vi "Argos_K_0v85.vi"(0 "PID 1 COM":refnum<visa-resource-name>="COM1", 1 "Setpoint\n START":bool, 2 "Write to File":bool, 3 "SP 1 input (°C)":dbl=20.0 min=0.0 max=1300.0, 4 "Intervall (s)":u32=1 max=600, 5 "Write/\nRead":bool=TRUE, 6 "Delay (ms)":u32=500 min=100 max=600000, 7 "Auto Tune":bool, 9 "Standby":bool, 11 "Reset\nSTOP":bool, 12 "ON":bool=TRUE caption="OFF", 13 "Get Values":bool, 15 "File Path":path) -> (8 "(°C)":dbl format="%#.3f", 14 "SP 1 is (°C)":dbl)   [LabVIEW 2013]
doc: "1. Verwendung\n\nDas Programm dient der Steuerung und Abfrage des Thermocontrollers I3252 und dem Auslesen von zwei VC 840 Messgeräten und einem Druckmessgerät Pfeiffer Single Gauge. \nDie Messgeräte werden Standardmäßig ausgelesen und erst nach Betätigung des Schalters \"Write to File\" in einer Textdatei abgespeichert. Das Eingabefeld \"Intervall\" legt den Abstand der Messpunkte fest.\nDer Setpoint für den Thermocontroller wird erst nach Betätigung des Tasters \"Setpoint START\" übernommen und angesteuert. Er wird ind den EEPROM des Gerätes geschrieben. Die Regelung kann mit Hilfe des Schalters \"Standby\" unterbrochen werden. Durch den Taster \"Reset STOPP\" kann der Setpoint aus dem EEPROM gelöscht werden.\nDie Eingabeflächen \"Constant\" und \"Thickness\" dienen der Berechnung des spezifischen Widerstands.\nDie Eingabeflächen \"User\" und \"Sample\" werden in den Header der Textdatei übernommen.\nDer Indikator \"File Path\" zeigt den aktuellen Speicherort der Textdatei an. Dieser wird nach ausschalten des Schalters \"Write to File\" gelöscht. Bei erneuten Schreiben muss ein neuer Speicherort gewählt werden. Bei Wahl desselben Speicherorts werden sämtliche bereits gespeicherte Daten gelöscht.\n\n\n2. Erläuterungen zum Blockdiagramm\n2.1 äußere Sequenz\nDie äußerte Sequenz besteht aus fünf Frames. Der erste dient der Initialisierung der Ports. Der zweite dient als Verzögerung um dem Programm genug Zeit zu geben die Ports zu öffnen. Jedoch senden die beiden VC 840 bereits Informationen an den Computer die in einem Puffer zwischengespeichert werden. Im dritten Frame wird dieser Puffer geleert. Somit kommt es zu keinem Framing Error. Desweiteren wird in diesem Frame die Startzeit der Messungen genommen. Im vierten Frame wird die eigentliche Messung und Verarbeitung der Daten durchgeführt. Die while-Schleife wird nur durch Auftreten eines Fehlers oder durch Betätigung des Stopbuttons auf dem Front Panel in der oberen linken Ecke unterbrochen. Im fünften und letzten Frame werden die Ports wieder geschlossen und beim Auftreten eines Fehlers wird das Programm automatisch gestoppt. Falls kein Fehler auftritt wird die Sequenz von vorne abgearbeitet.\n\n2.2 while-Schleife und innere Sequenz\n2.2.1 \"Event Structure\"\n2.2.1.1 Allgemein\nDer erste Frame beinhaltet ein \"Event Structure\". Dieser reagiert auf insgesamt elf verschiedene Ereignisse. Falls keines dieser Ereignisse auftreten sollte, warte die Struktur eine Millisekunde bevor die \"Event Structure\" verlassen wird. Die übrigen Ereignisse treten ein, wenn der entsprechende Kontroller eine Werteänderung erfährt.\n\n2.2.1.2 Event: Setpoint\nDieser Case besteht von außen nach innen aus einer Stacked Sequence, einer for-Loop und einer Flat Sequence die wiederum zwei \"Case Structures\" enthält. Als erstes wird bei dem Schalter \"Setpoint START\" der Blinkmodus aktiviert und bei dem Schalter \"Read Temperature\" deaktiviert. Danach folgt das eigentliche setzen des Temperatursollwerts. In der ersten Iteration wird dem Controller I3252 ein Schreibbefehl gesendet. Theoretisch kann der Setpoint in den RAM oder in den EEPROM geschrieben werden. Diese Auswahl erfolgt mit Hilfe des Schalters \"RAM\". Da das Schreiben in den RAM -Speicher aber aus diversen Gründen nicht erwünscht ist, wurde es nicht implementiert. Eine nachträgliche Implementierung ist aber leicht möglich, in dem die untere String-Konstante \"*P012\" durch \"*W012\" ersetzt wird. An diesem Befehl wird eine fünfstellige Hexadezimalzahl angehängt, die den Sollwert wiedergibt. Der Sollwert wird vorher mit zehn multipliziert, da das Komma standardmäßig nach der ersten Ziffer festgesetzt wurde (Bsp.: 800 wird gesendet um 80 einzustellen). Dieser Befehlsstrang wird an das Gerät mittels des SubVIs \"Comm_Interface\", auf welches später noch näher eingegangen wird, weitergegeben. Der durch das Gerät zurückgegebene String wird nicht verarbeitet.\nDie zweite Iteration dient dem Auslesen des eingestellten Sollwertes. Wahlweise kann der RAM- oder der EEPROM-Speicher ausgelesen werden. Die eigentliche Verarbeitung des Ausgabestrings erfolgt durch das SubVI \"Edit Setpoint\".\nDie Implementierung zur Einstellung des zweiten Setpoints erfolgt durch kopieren der ersten beiden Fälle und ersetzen der \"1\" im Befehf durch eine \"2\" (Bsp.: \"*P012\" zu \"*P022\"). Es darf aber nicht vergessen werden, dass dann ebenfalls die Anzahl der Iterationen angepasst werden muss.\nAls letztes wird der Blinkmodus des Schalters \"Setpoint START\" wieder deaktiviert.\n\n2.2.1.3 Event: Standby\nDieses Ereignis aktiviert bzw. deaktiviert als erstes den Blinckmodus des entsprechenden Schalters und sendet danach den Befehl zum aktivieren (\"*D03\") oder zum deaktivieren (\"*E03\") des Standbymodus an den Thermocontroller.\n\n2.2.1.4 Event: Set Command \nDer in das Feld \"Command shall be\" eingegebene Befehl wird an den Thermocontroller übermittlet. Die korrekte Form des Befehls ist im \"Communication Manuel\" nachzuschlagen. Das \"*\"-Zeichen wurde allerdings schon implementiert und muss somit nicht mit eingegeben werden.\n\n2.2.1.5 Event: Reset\nIn der ersten Iteration wird der Reset-Befehl an den Thermocontroller gesendet. In Folge wird der gesamte EEPROM-Speicher gelöscht. Deshalb wird in der zweiten Iteration der Setpoint aktualisiert. Dieser Befehl hat keinen Einfluss auf den RAM-Speicher. Die anschließende Wartezeit ist auf vier Sekunden festgesetzt und wurde empirisch ermittelt. Diese Zeit benötigt das Gerät um den Reset durchzuführen und für die Kommunikation wieder zur Verfügung zu stehen.\n\n2.2.1.6 Event: Auto Tune\nEs ist festgeschrieben, dass der Setpoint für die \"Auto Tune\"-Funktion wenigstens 20°C über der aktuellen Temperatur liegt. Deshalb wird zunächst der aktuelle Temperaturwert ausgelesen. Im zweiten Schritt werden zu diesem Wert zwanzig addiert und der Setpoint wird in den RAM-Speicher geschrieben. Das Schreiben in diesen Speicher ist nötig, da die \"Auto Tune\"-Funktion\" erst nach einem Reset startet. Im dritten Schritt wird der eigentliche Befehl für den \"Auto Tune\" gesendet (siehe dazu \"Communication Manuel\" S.27). Als vierte und letzte Iteration der for-Schleife folgt der bereits erwähnte Reset-Befehl. Der Temperatursollwert, der im RAM-Speicher eingetragen ist, muss zum Schluss wieder auf 0°C gesetzt werden. Die Zeit für die Ausführung des \"Auto Tune\"-Befehls wurde empirisch ermittelt und 45 s festgesetzt.\n\n2.2.1.7 Event: Write LOW/HI\nDieses Ereignis setzt die am Analogausgang anliegende Spannung fest. Normalerweise beträgt dieser Spannungswert 0-10 V. Das angeschlossene Netzteil verträgt aber maximal nur 2,3 V. Aus diesem Grund wird der \"%HIGH\" auf 23 gesetzt. Somit beträgt die maximal anliegende Spannung nur noch 23% von der maximal möglichen, d.h 2,3V. Ein niedrigerer Wert ist jederzeit möglich, genauso wie ein höherer für den Parameter \"%LOW\". Diese werden zunächst nacheinander in den RAM-Speicher geschrieben und anschließend wieder ausgelesen.\n\n2.2.1.8 Event: Set PID\nDie Werte für den PID-Regler können sowohl mit Hilfe der \"Auto Tune\"-Funktion, als auch manuell eingestellt werden. Es wird wiederum zwischen dem Schreiben in den RAM- und dem EEPROM-Speicher unterschieden. Zunächst werden die Werte für \"P\", \"I\" und \"D\", in dieser Reihenfolge, gesetzt und danach die aktuellen Werte ausgelesen.\n\n2.2.1.9 Event: Get Values\nDieses Ereignis hat zur Folge, dass die Werte für \"P\", \"I\", \"D\", \"%LOW\", \"%HIGH\" und des Setpoints wahlweise aus dem RAM- oder EEPROM-Speicher gelesen werden. Die aktuellen Werte werden nicht nur in die entsprechenden Anzeigefelder übernommen, sondern auch in die entsprechenden Eingabefelder, mit Ausnahme des Temperatursollwerts. \n\n2.2.1.10 Event: RAM\nPrinzipiell kann zwischen dem Schreiben in den RAM- oder EEPROM-Speicher des Thermocontrollers gewählt werden. Die entsprechende Schalterposition auf dem Frontpanel zeigt den aktuell verwendeten Speicher an. Die Anzeigewerte werden bei jedem Umschalten aktualisiert und sind im entsprechenden Speicher eingetragen. Die Implementierung ist identisch mit der des Ereignisses \"Get Values\". Es gilt zu beachten, dass die Werte für \"%LOW\" und \"%HIGH\" nur in den RAM-Speicher geschrieben werden können und somit auch nur aus diesem ausgelesen werden können.\n\n2.2.1.11 Event: Set Gauge to Zero\nMit Hilfe der SubVIs \"Get Pressure\" und \"Offset Display\" werden die Werte für den alten und den neuen Offset und der durch den zweiten Drucksensor ermittelt Druck ermittelt. \n\n2.2.1.12 Event: Write to File\nSollte der Schalter \"Write to File\" aktiviert werden, d.h. Schalterposition oben, so wird zunächst durch das SubVI \"Header\" ein Header für die unter \"File Path\" definierte Datei angelegt. Alle Werte, die bereits in der entsprechenden Datei stehen, werden dabei gelöscht.\n\n2.2.2 \"Timed Structures\"\nIm dritten Frame der inneren Sequenz werden die Werte für Zeitpunkt, Temperatur, Spannung, Strom und Druck ermittelt. Damit die Werte zum gleichen Zeitpunkt aufgenommen werden, werden \"Timed Sequences\" eingesetzt. Mit dem entsprechenden Schalter auf dem Front Panel unter dem Tab \"Settings\" kann gewählt werden, ob das entsprechende Gerät ausgelesen werden soll oder nicht. Die einzelnen Sequenzen werden parallel abgearbeitet, womit die Prozesszeit von diesem Frame durch der zeitintensivsten Sequenz abhängt. Dies ist in aller Regel das Auslesen der Temperatur, da ein \"Delay\" von 500 ms oder größer benötigt wird, um den Controller ordentlich ansprechen zu können.\nDie Systemzeit wird durch das SubVI \"System Time in Seconds\" in Sekunden umgerechnet und der in dem Parameter \"Starttime\" gespeicherte Wert wird abgezogen. Somit werden die Sekunden seit dem Start des Programms gezählt.\n\n2.2.3 restlichen Frames\nIm zweiten Frame wird das Intervall zwischen den einzelnen Messwerten festgelegt. Dabei wird der Wert des Parameters \"Delay\" abgezogen. Dieser Wert beträgt im Normalfall 500 ms und ist somit nicht vernachlääsigbar.\nDer Vierte Frame beinhaltet die Umrechnung des Temperatur-Strings in einen Temperaturwert durch das SubVI \"Edit Tmperature\", die Berechnung des spezifischen Widerstands durch das SubVI \"Resistivity Calculation\" und die Überprüfung des Druckwerts. Auch werden die neu gewonnen Werte in das entsprechende Shift-Register übernommen. Falls der Druckwert einen in dem Parameter \"Pressure Limit (mbar)\" festgelegten Grenzwert überschreiten sollte, wird der Thermocontroller automatisch in den Standby-Modus versetzt. Des Weiteren wird der Schalter \"Standby\" solange gesperrt, wie der Druck oberhalb des Grenzwertes liegt. Wenn der Druck wieder unter den Grenzwert gesunken ist, wird der Standby-Befehl nicht automatisch aufgehoben, sondern muss vom Benutzer durch Betätigung des entsprechenden Schalters gegeben werden.\nIm fünften Frame werden die Diagramme erstellt. Dabei wird jedes Mal von neuem das gesamte Shift-Register als Graph dargestellt. Weiterhin werden die Messwerte in ein 1D-Array geschrieben.\nDer sechste und letzte Frame beinhaltet den eigentlich Schreibvorgang der Messwerte in eine Textdatei und die Überprüfung ob ein Fehler vorliegt.\n\n2.3 SubVIs\n2.3.1 Allgemein\nDie SubVIs für die Messgeräte VC840 und das Druckmessgerät wurden aus anderen Quellen übernommen. \n\n2.3.2 \"Header\"\nIn den Header wird zunächst das aktuelle Datum und die aktuelle Zeit übernommen. Die ausgewählte Datei wird dabei überschrieben. Danach wird der Name des Benutzers und der Probe übernommen. Zum Schluss werden die Einheiten in einer Reihe, durch einen Tabulator getrennt, in den Header geschrieben.\n\n2.3.3 \"I3252 Comm Interface\"\nDieses VI stellt die Kommunikation mit dem Thermocontroller her und gibt den Ausgabe-String zurück.\n\n2.3.4 \"I3252 Edit Setpoint\"\nIm Ausgabe-String vom Thermocontroller ist an der vierten Stelle die Stelle des Dezimalpunktes verschlüsselt. Dieses Hexadezimalzahl wird herausgefiltert und an ein \"ENUM Controller\" übergeben. Dieser weist der Hexadezimalzahl eine Nummer zu, mit welcher ein Wert aus einem Array entnommen wird. Dieser Wert dient als Quotient. Der tatsächliche Wert kann somit errechnet werden.\n\n2.3.5 \"I3252 Edit Temperature\"\nDer Temperatur-String, der vom Thermocontroller zurückgegeben wird, wird in eine Dezimalzahl umgewandelt. Manchmal kommt es aus zu Dropouts, die durch dieses Programm herausgefiltert werden. Der letzte Wert wird dabei in einer \"Feedback Node\" gehalten unter der Annahme, dass sich der Temperaturwert nicht sprunghaft ändert.\n\n2.3.6 \"Resistivity Calculation\"\nDer spezifische Widerstand wird nach folgender Formel ausgerechnet. Dabei entspricht t der Dicke der Probe und C ist eine Konstante.\nrho=C*pi*t*U/(ln( 2)*I)\n\n2.3.7 \"System Time in Seconds\"\nZunächst wird die aktuelle Systemzeit ausgelesen. Danach wird diese in Stunden, Minuten und Sekunden aufgeteilt, alles in Sekunden umgerechnet und letztendlich addiert."
uses:
  <vilib>/Platform/TimedLoop/XDataNode/timing_clust.ctl
  <vilib>/Platform/TimedLoop/XDataNode/nitl_modes.ctl
  <vilib>/Platform/TimedLoop/XDataNode/wakeup.ctl
  <vilib>/Instr/_visa.llb/VISA Configure Serial Port (Instr).vi
  <vilib>/Platform/TimedLoop/scheduler/LVUserAPI/_suppVIs/Create_1kHz_TSource.vi
  <vilib>/Utility/file.llb/Write To Spreadsheet File (DBL).vi
  <vilib>/Platform/TimedLoop/XDataNode/XDataNode.xnode
  <vilib>/Platform/TimedLoop/XDataNode/XDNodeRunTimeDep.lvlib
  Argos0v7/Dependencies/Pfeiffer TPG261+262 Single+Dual Gauge/Dual Gauge.lvlib
panel:
  out "Thermocouple (Sample holder 1) 2":cluster{dbl[], dbl[]}(graph)
  out "(°C) 2":dbl format="%#.3f"
  out "appended array":dbl[](array[numeric])
  in  "Tab Control":T1(tab)
  out "SP 2 is (°C)":dbl
  in  "SP 2 input (°C)":dbl=20.0 min=0.0 max=1300.0
  in  "Standby\n2":bool
  in  "Setpoint\n START\n2":bool
  out "Pirani (VVP1 Scroll)":cluster{dbl[], dbl[]}(graph)
  in  "Thickness (nm)":dbl min=0.0
  in  "4PP constant":dbl min=0.0 max=5.0
  in  "Sample":string
  in  "User":string
  out "Thermocouple (Sample holder 1)":cluster{dbl[], dbl[]}(graph)
  out "current time (s)":dbl
  out "data logger intervall (s)":dbl
  out "loop time (s)":dbl
  in  "stop":bool
  out "CMR275 Baratron":cluster{dbl[], dbl[]}(graph)
  out "Pressure Baratron 2":dbl format="%#_4e"
  out "PKR251 FullRange":cluster{dbl[], dbl[]}(graph)
  out "Pressure FullRange 2":dbl format="%#_3e"
  out "Pressure Pirani 2":dbl format="%#_3e"
  in  "Reset\nSTOP 2":bool
  out "Pressure OpenPort":cluster{dbl[], dbl[]}(graph)
  out "Pressure OpenPort2":dbl caption="current"
  out "% HIGH Istwert 2":u32
  out "% LOW Istwert 2":u32
  in  "% High Sollwert 2":u32=23 max=24
  in  "% LOW Sollwert 2":u32 max=25
  in  "RAM 2":bool=TRUE caption="EEPROM"
  out "D (Rate) IstWert 2":u32
  out "I ( Reset1) Istwert 2":u32
  out "P (PB1) Istwert 2":u32 caption="actual value"
  in  "D (Rate) Sollwert 2":u32 max=3999
  in  "I ( Reset1) Sollwert 2":u32 max=3999
  in  "P (PB1) Sollwert 2":u32 caption="set value" max=9999
  in  "ON 2":bool=TRUE caption="OFF"
  in  "PID 2 COM":refnum<visa-resource-name>="COM1"
  in  "Baud Rate 2":u32=9600
  in  "Data Bits 2":u16=7 min=5 max=8 step=1
  in  "Parity 2":u16(ring)=1 items=["None", "Odd", "Even", "Mark", "Space"]
  in  "Stop Bits 2":u16(ring)=10 items=["1.0"=10, "1.5"=15, "2.0"=20]
  in  "Flow Control 2":u16(ring) items=["None"=0, "XON/XOFF"=1, "RTS/CTS"=2, "DTR/DSR"=4]
  in  "Delay (ms) 2":u32=500 min=100 max=600000
  in  "Write/\nRead \n\n2":bool=TRUE
  out "status 2":bool caption="Status"
  out "code 2":i32 caption="Code"
  out "code":i32 caption="Code"
  out "status":bool caption="Status"
  in  "Set Gauge to Zero":bool
  out "Status Gauge 1#2":i32(ring) items=["data OK", "underrange", "overrange", "sensor error", "sensor off", "no sensor", "ID error"]
  out "Pressure Gauge 1#2":dbl format="%.3e"
  out "Pressure Gauge 1#1":dbl format="%.3e"
  out "Status Gauge 1#1":i32(ring) items=["data OK", "underrange", "overrange", "sensor error", "sensor off", "no sensor", "ID error"]
  in  "TPG 1 COM":refnum<visa-resource-name>="COM5"
  in  "Pressure Limit (mbar)":dbl=1.0 min=0.0 max=1100.0
  out "Current Offset (mbar)":dbl
  in  "ON (TPG 2)":bool=TRUE caption="OFF"
  in  "ON (TPG 1)":bool=TRUE caption="OFF"
  in  "ON":bool caption="OFF"
  in  "VC 840 2":refnum<visa-resource-name>="COM7"
  out "Reading 2":dbl format="%_4f"
  out "Mode 2":enum16{"?", "Diode", "Beep", "DC", "AC"}(ring)
  out "Unit 2":string
  in  "VC 840 1":refnum<visa-resource-name>="COM7"
  out "Reading 1":dbl format="%_4f"
  out "Mode 1":enum16{"?", "Diode", "Beep", "DC", "AC"}(ring)
  out "Unit 1":string
  out "Status 1":T2
  out "Status 2":T2
  in  "ON":bool caption="OFF"
  out "% HIGH Istwert":u32
  out "% LOW Istwert":u32
  in  "% High Sollwert":u32=23 max=24
  in  "% LOW Sollwert":u32 max=25
  in  "RAM":bool=TRUE caption="EEPROM"
  out "D (Rate) IstWert":u32
  out "I ( Reset1) Istwert":u32
  out "P (PB1) Istwert":u32 caption="actual value"
  in  "D (Rate) Sollwert":u32 max=3999
  in  "I ( Reset1) Sollwert":u32 max=3999
  in  "P (PB1) Sollwert":u32 caption="set value" max=9999
  in  "Set Command":bool
  in  "Set PID":bool
  in  "Write LOW/HI":bool
  in  "Flow Control":u16(ring) items=["None"=0, "XON/XOFF"=1, "RTS/CTS"=2, "DTR/DSR"=4]
  in  "Stop Bits":u16(ring)=10 items=["1.0"=10, "1.5"=15, "2.0"=20]
  in  "Parity":u16(ring)=1 items=["None", "Odd", "Even", "Mark", "Space"]
  in  "Data Bits":u16=7 min=5 max=8 step=1
  in  "Baud Rate":u32=9600
  out "Command output":string
  in  "Command input":string
  in  "TPG 2 COM":refnum<visa-resource-name>="COM6"
  out "Pressure Gauge 2#2":dbl format="%.3e"
  out "Pressure Gauge 2#1":dbl format="%.3e"
  out "Status Gauge 2#2":i32(ring) items=["data OK", "underrange", "overrange", "sensor error", "sensor off", "no sensor", "ID error"]
  out "Status Gauge 2#1":i32(ring) items=["data OK", "underrange", "overrange", "sensor error", "sensor off", "no sensor", "ID error"]
  out "Command output 2":string
  in  "Command input 2":string
  in  "Set Command\n\n 2":bool
  in  "Auto Tune 2":bool
  in  "Set PID 2":bool
  in  "Write LOW/HI 2":bool
  in  "Get Values 2":bool
  out "Current":cluster{dbl[], dbl[]}(graph)
  out "Voltage":cluster{dbl[], dbl[]}(graph)
  out "Voltage (V)":dbl format="%.4e"
  out "Current (A)":dbl format="%.4e"
  out "Resistivity":cluster{dbl[], dbl[]}(graph)
  out "Resistivity (Ohm*cm)":dbl format="%.3e"
  # "PID 1"
  # "set \nvalue"
  # "actual \nvalue"
  # "T (°C)"
  # "PID 2"
  # "mbar"
  # "Set \nValue\n2"
  # "Actual \nvalue 2"
  # "T (°C)"
  # "mbar"
  # "mbar"
  # "mbar"
  # "Pressure Measurement \n(Pfeiffer TPG261)"
  # "PID Controller (Omega Newport i3252)"
  # "PID Controller 2 (Omega Newport i3252)"
  # "limit (mbar)"
  # "P"
  # "I"
  # "D"
  # "% Low"
  # "% High"
  # "Multimeter\n#1 (VC 840)"
  # "Multimeter\n#2 (VC 840)"
  # "P"
  # "I"
  # "D"
  # "% Low"
  # "% High"
  # "Authors:  Daniel Schuster (sir-dan@web.de)\n                 Steffen Cornelius (s.cornelius@hzdr.de)\n                 Nico Spahn (x)\n\n                 premade SubVIs for readout of Pfeiffer gauge and VC840 Multimeters were used\n                 SubVI \"I3252_Comm_Interface\" is based on a modified Labview example\n\nRelease:  v1.0    \n\nVersion History:\n\nv1.1  -    28.06.2011\n             - Format des Files geändert von %.3f auf %g\n             - maximale Eingabewerte für PID begrenzt\nv1.2  -    12.07.2011\n             - Anzeige p,rho, U, V auf Scientific geändert\n             - y-Achse p,rho auf Log geändert\n             - numerische Zeitanzeige hinzugefügt\n             - 4PP Constant: pi/ln(2)=4,532 set as the default value\nv1.3  -    25.07.2011\n             - Zeitvariable auf EXT geändert, um Sprünge in Diagrammen loszuwerden\nv1.4  -   27.07.2011\n             - ALLE Variablen auf DBL zurückgesetzt wegen Formatierungsproblem im File\n             - Zeitberechnung neu gemacht (Tick count differenzen) -> Zeitsprünge korrigiert ?\n             - Delay/Intervall überarbeitet\nv1.5  -   05.12.2012\n                - Austausch der alten Pfeifer SubvIs durch neue -> nun alle 4 Kanäle des DualGauge\n                                                                                                         Controllers gleichzeitig auslesbar\n                - neue Pfeiffer SubVIs verwendet in Druckwertauslesung und Offset Berechnung des Baratron\n                  Druckes (COM5 Sensor1)\n                - Neuarragement des GUI -> FullRange und Baratron neben Temperatur auf Haupseite zu sehen\n                                                                   Pirani und OpenPort auf Meas.2 zu sehen\n                                                                   Diagnose Seite umfasst nun auch Widerstandsdiagramm\n                - Änderungen der Settingseite -> nun alle 4 Drucksensoren mit aktuellem Messwert und Gerätestatus\n                                                                           zu sehen\n                - The readout of the PID-Temperature Controller and the VC840 Multimeters was not modified\nv1.73  -  18.10.2013\n                - Layout Änderungen\nv.1.8   -  19.01.2014\n                - Änderung Layout Settings Tab\n                - Trennung der beiden TPG Dual Gauge Controls\n                -"
  # "Version 1.73    - last change 18.10.2013"
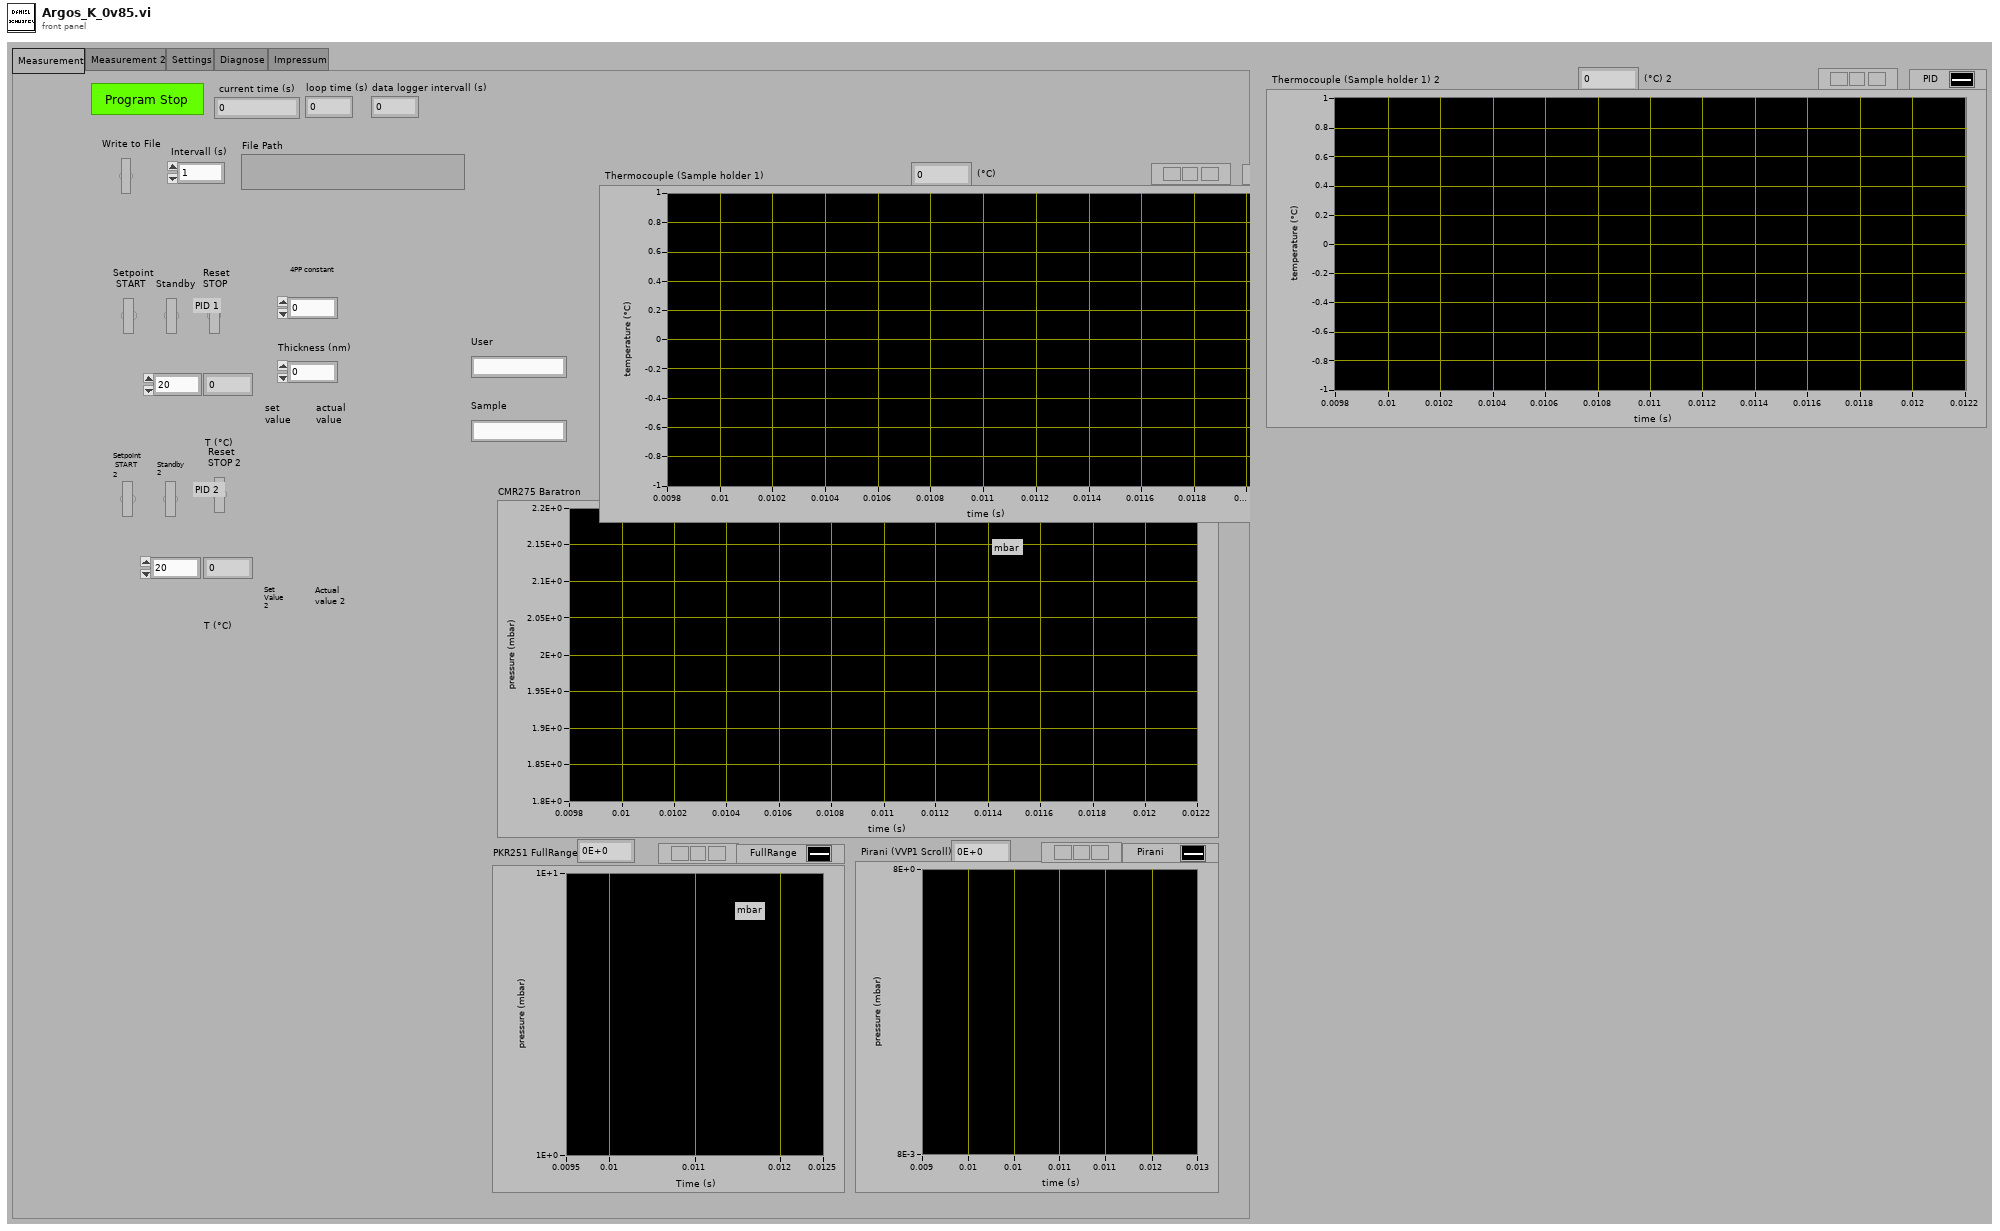
[diagram p1: front panel]
types:
  T1 = enum32{"Measurement", "Measurement 2", "Settings", "Diagnose", "Impressum"}
  T2 = cluster{"Low Bat":bool, "Auto":bool, "Delta":bool, "Hold":bool, "RS232":bool}
  T3 = typedef "XDNodeRunTimeDep.lvlib/timing_clust.ctl" = cluster{"Expected End [f-1]":u64, "Actual End [f-1]":u64, "Finished Late? [f-1]":bool, "Expected End [i-1]":u64, "Actual End [i-1]":u64, "Finished Late? [i-1]":bool, "Expected Start [i]":u64, "Actual Start [i]":u64, "Expected Start [f]":u64, "Actual Start [f]":u64, "Source Name":string, "Structure Name":string, "Period":i64, "Deadline":i64, "Offset":i64, "Start":i64, "Priority":i32, "Timeout":i32, "Mode":T4, "Wakeup Reason":T5, "Error":errorcluster, "Source Type":string, "Secondary Source Type":string, "Global End Time":u64, "Global Start Time":u64, "Frame Duration":u64, "Iteration Duration":u64, "Assigned CPU":i32, "I/O Scan Engine Mode":u32}
  T4 = typedef "XDNodeRunTimeDep.lvlib/nitl_modes.ctl" = enum32{"No Change", "Process missed periods, maintain original phase", "Discard missed periods, maintain original phase", "Process missed periods, ignore original phase", "Discard missed periods, ignore original phase"}
  T5 = typedef "XDNodeRunTimeDep.lvlib/wakeup.ctl" = enum32{"Normal", "Aborted", "Asynchronous wakeup", "Timing source error", "Timed loop error", "Timeout"}
  T6 = enum8{"Enabled", "Disabled", "Disabled and Grayed Out"}
  T7 = cluster{"VISA resource name out":refnum<visa-resource-name>, "error out":errorcluster, "Delay (ms)":u32, "Write/\nRead":bool}
  T8 = cluster{"VISA resource name out":refnum<visa-resource-name>, "error out":errorcluster, "Delay (ms) 2":u32, "Write/\nRead \n\n2":bool}
  T9 = cluster{"TPG 2 COM":refnum<visa-resource-name>, "error out":errorcluster}
  T10 = cluster{"COM out":refnum<visa-resource-name>, "Cluster (Ausgang)":errorcluster}
  T11 = cluster{"Pressure Gauge#1":dbl, "Pressure Gauge#2":dbl}
  T12 = cluster{"TPG 1 COM":refnum<visa-resource-name>, "error out":errorcluster}
  T13 = cluster{"COM out":refnum<visa-resource-name>, "error out":errorcluster, "COM out":refnum<visa-resource-name>, "error out":errorcluster}
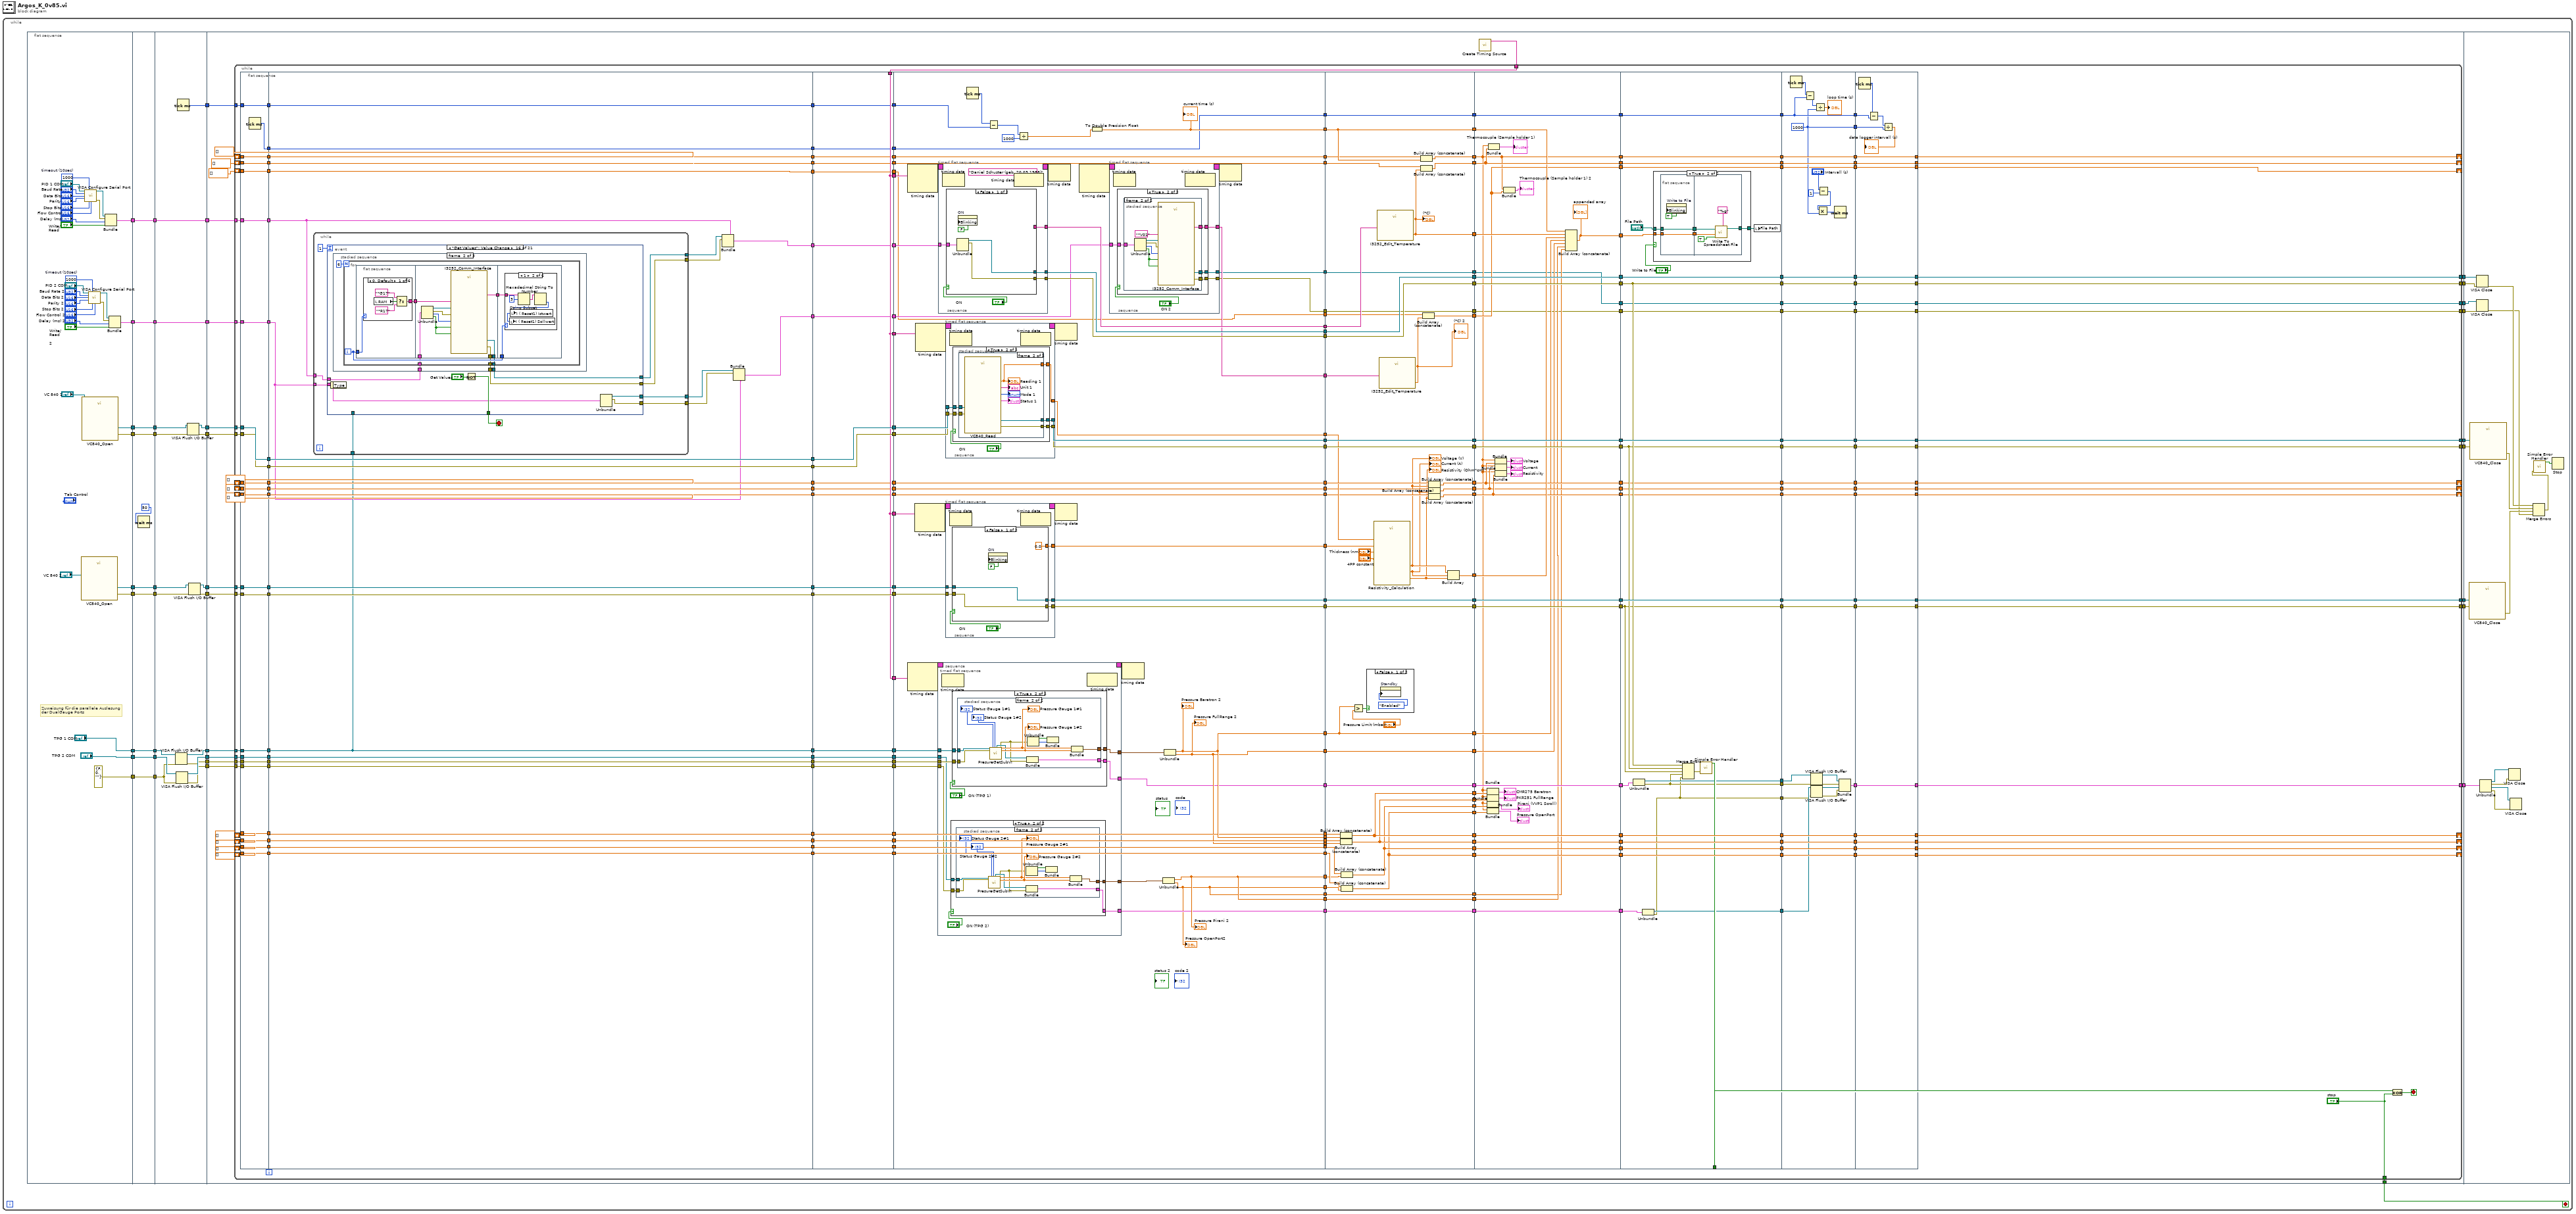
[diagram p0: block diagram]
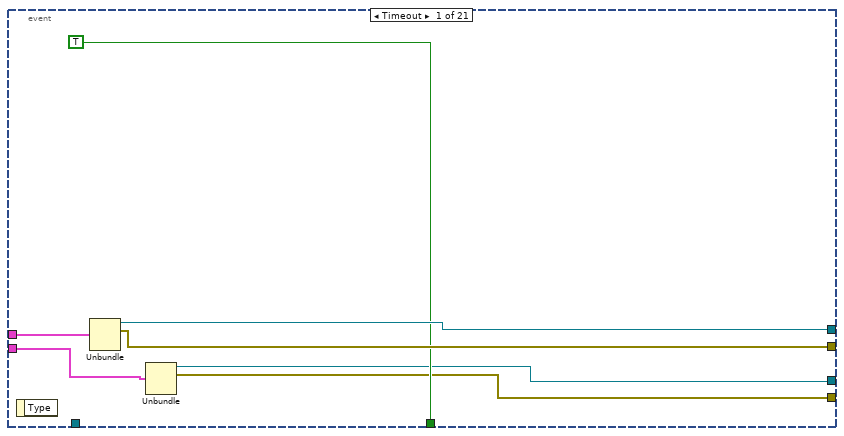
[diagram p2: hidden frame]
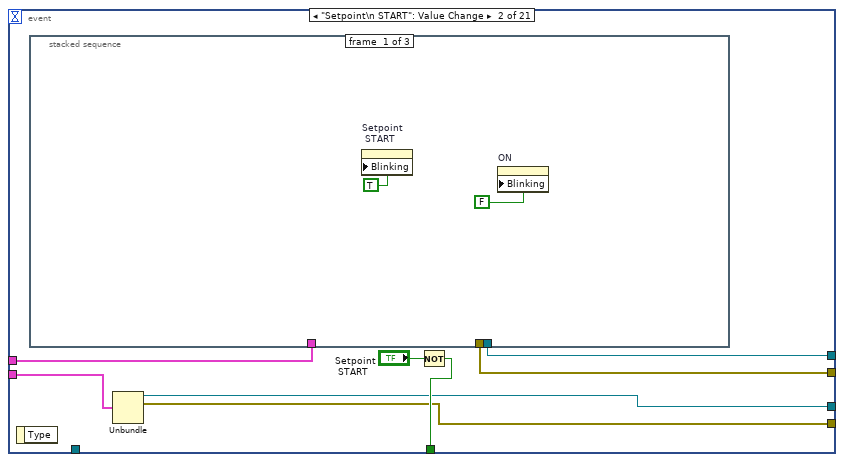
[diagram p3: hidden frame]
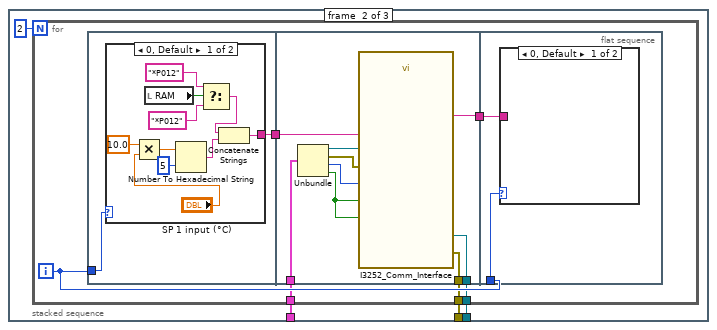
[diagram p4: hidden frame]
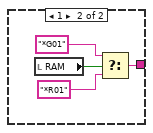
[diagram p5: hidden frame]
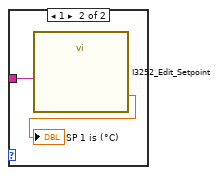
[diagram p6: hidden frame]
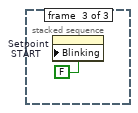
[diagram p7: hidden frame]
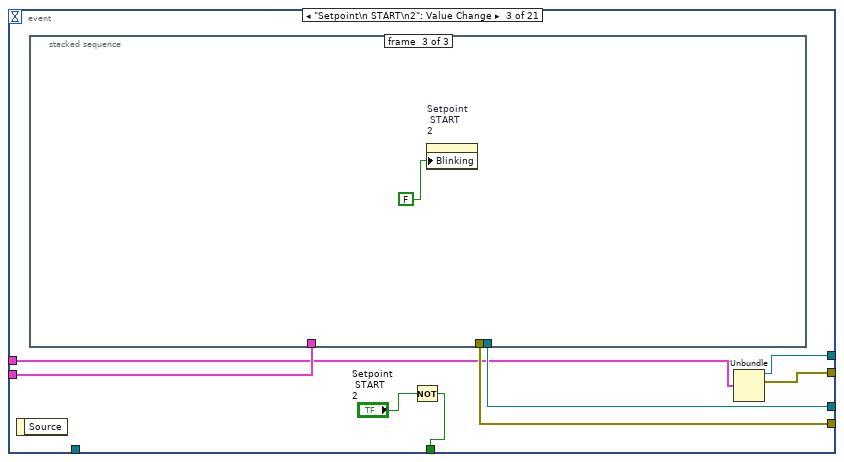
[diagram p8: hidden frame]
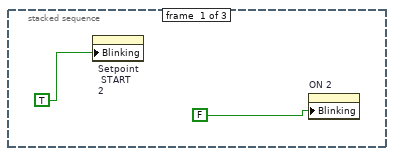
[diagram p9: hidden frame]
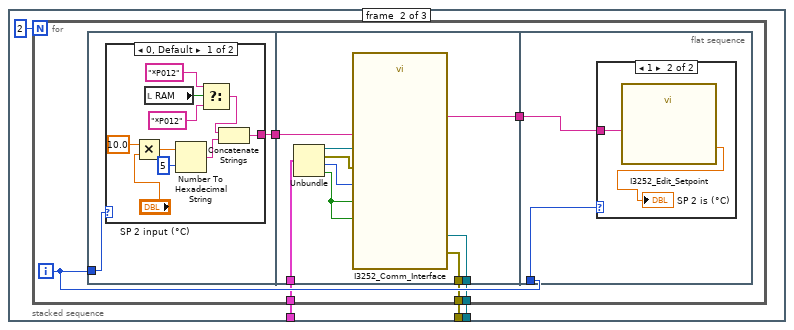
[diagram p10: hidden frame]
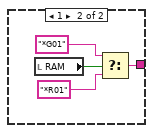
[diagram p11: hidden frame]
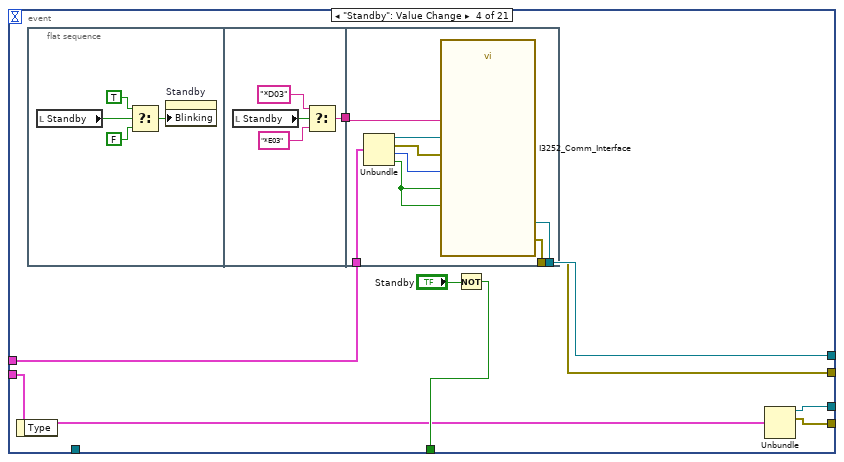
[diagram p13: hidden frame]
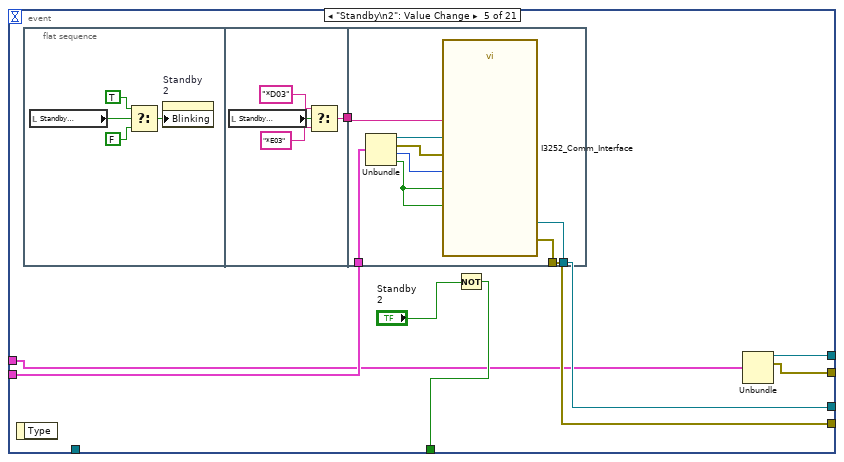
[diagram p14: hidden frame]
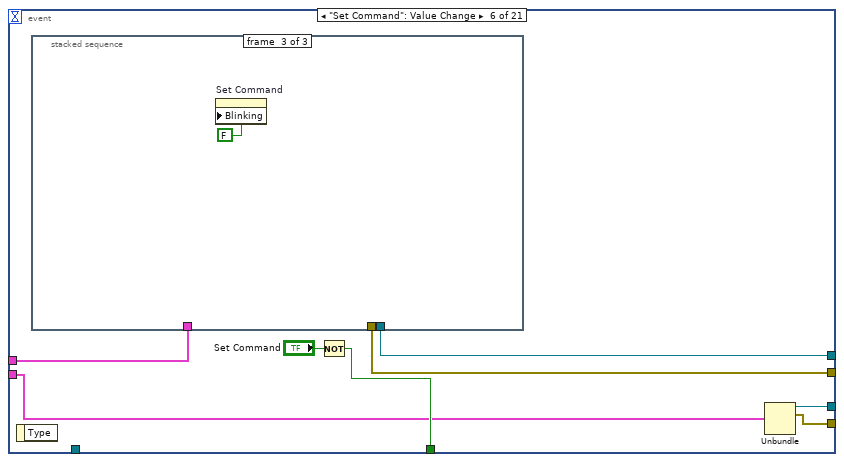
[diagram p15: hidden frame]
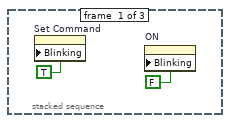
[diagram p16: hidden frame]
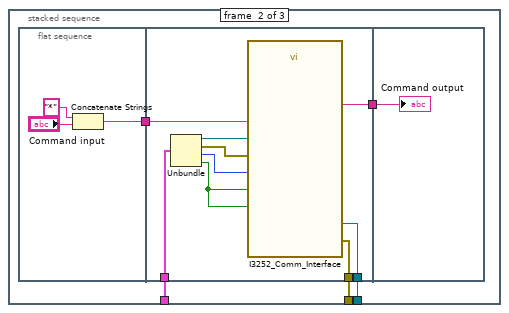
[diagram p17: hidden frame]
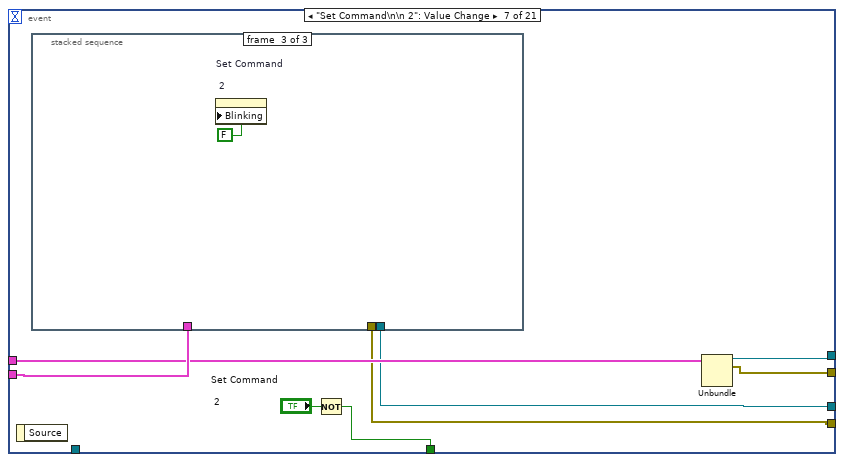
[diagram p18: hidden frame]
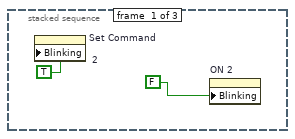
[diagram p19: hidden frame]
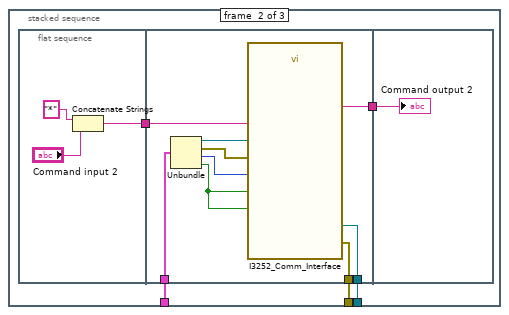
[diagram p20: hidden frame]
diagram:
  n1 = while {
    stop <- w11 stop-if-true
    n2 = flat-sequence {
      tunnel: [w71] -> w39
      tunnel: [w72] -> w38
      tunnel: [w57] -> w37
      tunnel: [w70] -> w36
      tunnel: [w69] -> w35
      tunnel: ["TPG 1 COM"] -> w34
      tunnel: ["TPG 2 COM"] -> w33
      tunnel: [errorcluster {"status"=FALSE, "code"=0, "source"=""} ("Fehler (Eingang)")] -> w8
      tunnel: [w40] -> w3
      tunnel: w39 -> [w82]
      tunnel: [w82] -> w32
      tunnel: w38 -> [w81]
      tunnel: [w81] -> w31
      tunnel: w37 -> [w80]
      tunnel: [w80] -> w30
      tunnel: w36 -> [w79]
      tunnel: [w79] -> w29
      tunnel: w35 -> [w78]
      tunnel: [w78] -> w28
      tunnel: [w76] -> w27
      tunnel: w34 -> [w76]
      tunnel: [w75] -> w26
      tunnel: w33 -> [w75]
      tunnel: [w74] -> w9
      tunnel: w8 -> [w74]
      tunnel: [w73] -> w4
      tunnel: w3 -> [w73]
      tunnel: w32 -> [w94]
      tunnel: [w93] -> w25
      tunnel: w31 -> [w95]
      tunnel: [w92] -> w24
      tunnel: w30 -> [w100]
      tunnel: [w100] -> w23
      tunnel: w29 -> [w97]
      tunnel: [w98] -> w22
      tunnel: w28 -> [w96]
      tunnel: [w99] -> w21
      tunnel: [w91] -> w20
      tunnel: [w89] -> w19
      tunnel: w27 -> [w90]
      tunnel: [w88] -> w18
      tunnel: w26 -> [w87]
      tunnel: w9 -> [w86]
      tunnel: [w85] -> w7
      tunnel: [w84] -> w6
      tunnel: [w83] -> w5
      tunnel: w4 -> [w83]
      tunnel: w25 -> [w132]
      tunnel: w24 -> [w131]
      tunnel: w23 -> [w130]
      tunnel: w22 -> [w128]
      tunnel: w21 -> [w127]
      tunnel: [w126] -> w17
      tunnel: [w125] -> w16
      tunnel: [w124] -> w15
      tunnel: [w123] -> w14
      tunnel: [w122] -> w13
      tunnel: [w121] -> w12
      tunnel: w20 -> [w115]
      tunnel: w19 -> [w114]
      tunnel: w18 -> [w113]
      tunnel: [w108] -> w11
      tunnel: [w107] -> w10
      tunnel: w7 -> [w106]
      tunnel: w6 -> [w105]
      tunnel: w5 -> [w104]
      tunnel: [w103] -> w2
      tunnel: [w102] -> w1
      tunnel: w17 -> [w1957]
      tunnel: w16 -> [w1956]
      tunnel: w15 -> [w1959]
      tunnel: w14 -> [w1958]
      tunnel: w13 -> [w1961]
      tunnel: w12 -> [w1960]
      tunnel: w10 -> [w1954]
      tunnel: w2 -> [w1949]
      tunnel: w1 -> [w1948]
      frame #0 {
        w41 = u32 1000  # timeout (10sec)
        w58 = u32 1000  # timeout (10sec)
        # "Zuweisung für die parallele Auslesung\nder DualGauge Ports"
        n3 = call "VC840_Open.vi"("VISA resource name"="VC 840 2") -> ("error out"=w69:errorcluster, "VISA resource name out"=w70:refnum<visa-resource-name>)  [unwired: 1 in, 8 out]
        n4 = call "VC840_Open.vi"("VISA resource name"="VC 840 1") -> ("error out"=w72:errorcluster, "VISA resource name out"=w71:refnum<visa-resource-name>)  [unwired: 1 in, 8 out]
        n5 = call-poly "VISA Configure Serial Port"("VISA resource name"="PID 1 COM", "timeout (10sec)"=w58, "baud rate (9600)"="Baud Rate", "data bits (8)"="Data Bits", "parity (0:none)"="Parity", "stop bits (10: 1 bit)"="Stop Bits", "flow control (0:none)"="Flow Control") -> ("VISA resource name out"=w67:refnum<visa-resource-name>, "error out"=w68:errorcluster)  [unwired: 2 in, 5 out]
        n6 = call-poly "VISA Configure Serial Port"("VISA resource name"="PID 2 COM", "timeout (10sec)"=w41, "baud rate (9600)"="Baud Rate 2", "data bits (8)"="Data Bits 2", "parity (0:none)"="Parity 2", "stop bits (10: 1 bit)"="Stop Bits 2", "flow control (0:none)"="Flow Control 2") -> ("VISA resource name out"=w50:refnum<visa-resource-name>, "error out"=w51:errorcluster)  [unwired: 2 in, 5 out]
        n7 = Bundle("VISA resource name out"=w67, "error out"=w68, "Delay (ms)"="Delay (ms)", "Write/\nRead"="Write/\nRead") -> (w57:T7)  [unwired: 1 in]
        n8 = Bundle("VISA resource name out"=w50, "error out"=w51, "Delay (ms) 2"="Delay (ms) 2", "Write/\nRead \n\n2"="Write/\nRead \n\n2") -> (w40:T8)  [unwired: 1 in]
      }
      frame #1 {
        n9 = Wait (ms)(milliseconds to wait=u32 50) -> ()  [unwired: 1 out]
      }
      frame #2 {
        n10 = VISA Flush I/O Buffer(VISA resource name=w90, error in (no error)=w86) -> (VISA resource name out=w89:refnum<visa-resource-name>, error out=w85:errorcluster)  [unwired: 1 in]
        n11 = VISA Flush I/O Buffer(VISA resource name=w87, error in (no error)=w86) -> (VISA resource name out=w88:refnum<visa-resource-name>, error out=w84:errorcluster)  [unwired: 1 in]
        n12 = Tick Count (ms)() -> (millisecond timer value=w91:u32)
        n13 = VISA Flush I/O Buffer(VISA resource name=w94, error in (no error)=w95) -> (VISA resource name out=w93:refnum<visa-resource-name>, error out=w92:errorcluster)  [unwired: 1 in]
        n14 = VISA Flush I/O Buffer(VISA resource name=w97, error in (no error)=w96) -> (VISA resource name out=w98:refnum<visa-resource-name>, error out=w99:errorcluster)  [unwired: 1 in]
      }
      frame #3 {
        n15 = call-poly <vilib>:"Create Timing Source.vi"() -> ("name (out)"=w129:string)  [unwired: 10 in, 1 out]
        n16 = while {
          tunnel: w132 -> [w378]
          tunnel: w131 -> [w377]
          tunnel: w130 -> [w376]
          tunnel: w129 -> [w369]
          tunnel: w128 -> [w362]
          tunnel: w127 -> [w361]
          tunnel: [w357] -> w126
          tunnel: [w356] -> w125
          tunnel: [w354] -> w124
          tunnel: [w352] -> w123
          tunnel: [w350] -> w122
          tunnel: [w348] -> w121
          shift-right: [w321] -> _
          shift-left: dbl[] [] -> [w326]
          shift-right: [w299] -> _
          shift-left: dbl[] [] -> [w334]
          shift-right: [w323] -> _
          shift-left: dbl[] [] -> [w330]
          shift-right: [w296] -> _
          shift-left: dbl[] [] -> [w333]
          shift-right: [w293] -> _
          shift-left: dbl[] [] -> [w332]
          tunnel: w115 -> [w287]
          tunnel: w114 -> [w243]
          tunnel: w113 -> [w239]
          shift-right: [w197] -> _
          shift-left: dbl[] [] -> [w227]
          shift-right: [w195] -> _
          shift-left: dbl[] [] -> [w225]
          shift-right: [w193] -> _
          shift-left: dbl[] [] -> [w223]
          shift-right: [w191] -> _
          shift-left: dbl[] [] -> [w221]
          tunnel: ["stop"] -> w108
          tunnel: [w185] -> w107
          tunnel: w106 -> [w180]
          tunnel: w105 -> [w178]
          tunnel: w104 -> [w158]
          shift-right: [w150] -> _
          shift-left: dbl[] [] -> [w148]
          tunnel: [w139] -> w103
          tunnel: [w133] -> w102
          stop <- w184 stop-if-true
          n17 = flat-sequence {
            tunnel: w287 -> [w390]
            tunnel: w326 -> [w391]
            tunnel: w330 -> [w392]
            tunnel: w332 -> [w393]
            tunnel: w333 -> [w394]
            tunnel: w334 -> [w395]
            tunnel: w361 -> [w396]
            tunnel: w362 -> [w397]
            tunnel: w376 -> [w398]
            tunnel: w377 -> [w399]
            tunnel: w378 -> [w400]
            tunnel: [w400] -> w286
            tunnel: [w399] -> w285
            tunnel: [w398] -> w284
            tunnel: [w397] -> w283
            tunnel: [w396] -> w282
            tunnel: [w395] -> w281
            tunnel: [w394] -> w280
            tunnel: [w393] -> w279
            tunnel: [w392] -> w278
            tunnel: [w391] -> w277
            tunnel: [w390] -> w276
            tunnel: [w389] -> w258
            tunnel: [w388] -> w244
            tunnel: w243 -> [w388]
            tunnel: [w387] -> w240
            tunnel: w239 -> [w387]
            tunnel: [w386] -> w228
            tunnel: w227 -> [w386]
            tunnel: [w385] -> w226
            tunnel: w225 -> [w385]
            tunnel: [w384] -> w224
            tunnel: w223 -> [w384]
            tunnel: [w383] -> w222
            tunnel: w221 -> [w383]
            tunnel: [w382] -> w181
            tunnel: w180 -> [w382]
            tunnel: [w381] -> w179
            tunnel: w178 -> [w381]
            tunnel: [w380] -> w159
            tunnel: w158 -> [w380]
            tunnel: [w379] -> w149
            tunnel: w148 -> [w379]
            tunnel: [w428] -> w375
            tunnel: [w427] -> w373
            tunnel: [w423] -> w371
            tunnel: [w422] -> w366
            tunnel: [w421] -> w364
            tunnel: [w420] -> w331
            tunnel: [w419] -> w327
            tunnel: [w418] -> w307
            tunnel: [w417] -> w304
            tunnel: [w416] -> w302
            tunnel: [w415] -> w288
            tunnel: w286 -> [w428]
            tunnel: w285 -> [w427]
            tunnel: w284 -> [w426]
            tunnel: w283 -> [w422]
            tunnel: w282 -> [w421]
            tunnel: w281 -> [w418]
            tunnel: w280 -> [w417]
            tunnel: w279 -> [w416]
            tunnel: w278 -> [w420]
            tunnel: w277 -> [w419]
            tunnel: w276 -> [w415]
            tunnel: [w414] -> w259
            tunnel: w258 -> [w414]
            tunnel: w244 -> [w412]
            tunnel: [w412] -> w241
            tunnel: w240 -> [w413]
            tunnel: [w413] -> w237
            tunnel: w228 -> [w411]
            tunnel: w226 -> [w410]
            tunnel: w224 -> [w409]
            tunnel: w222 -> [w408]
            tunnel: [w411] -> w220
            tunnel: [w410] -> w216
            tunnel: [w409] -> w213
            tunnel: [w408] -> w212
            tunnel: w181 -> [w407]
            tunnel: w179 -> [w406]
            tunnel: [w407] -> w176
            tunnel: [w406] -> w174
            tunnel: w159 -> [w402]
            tunnel: [w401] -> w156
            tunnel: w149 -> [w405]
            tunnel: [w405] -> w147
            tunnel: w375 -> [w1479]
            tunnel: [w1479] -> w374
            tunnel: w373 -> [w1478]
            tunnel: [w1478] -> w372
            tunnel: w371 -> [w1474]
            tunnel: [w1474] -> w370
            tunnel: w369 -> [w1475]
            tunnel: [w1475] -> w368
            tunnel: [w1475] -> w367
            tunnel: w366 -> [w1477]
            tunnel: [w1477] -> w365
            tunnel: w364 -> [w1476]
            tunnel: [w1476] -> w363
            tunnel: [w1475] -> w360
            tunnel: [w1475] -> w346
            tunnel: w331 -> [w1473]
            tunnel: [w1473] -> w329
            tunnel: w327 -> [w1472]
            tunnel: [w1472] -> w324
            tunnel: [w1471] -> w308
            tunnel: w307 -> [w1471]
            tunnel: [w1470] -> w305
            tunnel: w304 -> [w1470]
            tunnel: [w1469] -> w303
            tunnel: w302 -> [w1469]
            tunnel: [w1468] -> w289
            tunnel: w288 -> [w1468]
            tunnel: [w1467] -> w260
            tunnel: w259 -> [w1467]
            tunnel: [w1466] -> w242
            tunnel: w241 -> [w1466]
            tunnel: [w1465] -> w238
            tunnel: w237 -> [w1465]
            tunnel: w220 -> [w1464]
            tunnel: [w1464] -> w219
            tunnel: [w1463] -> w217
            tunnel: w216 -> [w1463]
            tunnel: [w1462] -> w215
            tunnel: w213 -> [w1462]
            tunnel: w212 -> [w1461]
            tunnel: [w1461] -> w211
            tunnel: [w1460] -> w177
            tunnel: w176 -> [w1460]
            tunnel: [w1459] -> w175
            tunnel: w174 -> [w1459]
            tunnel: [w1458] -> w157
            tunnel: w156 -> [w1458]
            tunnel: w147 -> [w1457]
            tunnel: [w1457] -> w146
            tunnel: [w1509] -> w345
            tunnel: w374 -> [w1538]
            tunnel: w372 -> [w1537]
            tunnel: w370 -> [w1534]
            tunnel: w368 -> [w1533]
            tunnel: w367 -> [w1532]
            tunnel: w365 -> [w1522]
            tunnel: w363 -> [w1521]
            tunnel: w360 -> [w1523]
            tunnel: [w1519] -> w344
            tunnel: [w1520] -> w343
            tunnel: [w1531] -> w342
            tunnel: [w1530] -> w341
            tunnel: [w1529] -> w340
            tunnel: [w1528] -> w339
            tunnel: w346 -> [w1518]
            tunnel: [w1517] -> w338
            tunnel: [w1516] -> w337
            tunnel: [w1500] -> w336
            tunnel: [w1515] -> w335
            tunnel: w329 -> [w1514]
            tunnel: [w1514] -> w328
            tunnel: [w1513] -> w325
            tunnel: w324 -> [w1513]
            tunnel: w308 -> [w1512]
            tunnel: [w1512] -> w306
            tunnel: w305 -> [w1511]
            tunnel: w303 -> [w1510]
            tunnel: [w1511] -> w301
            tunnel: [w1510] -> w300
            tunnel: w289 -> [w1508]
            tunnel: [w1504] -> w261
            tunnel: w260 -> [w1504]
            tunnel: w242 -> [w1502]
            tunnel: w238 -> [w1501]
            tunnel: [w1495] -> w236
            tunnel: [w1500] -> w235
            tunnel: [w1498] -> w234
            tunnel: [w1496] -> w233
            tunnel: w219 -> [w1499]
            tunnel: [w1499] -> w218
            tunnel: w217 -> [w1498]
            tunnel: w215 -> [w1497]
            tunnel: [w1497] -> w214
            tunnel: w211 -> [w1496]
            tunnel: [w1495] -> w189
            tunnel: [w1494] -> w186
            tunnel: w177 -> [w1493]
            tunnel: w175 -> [w1492]
            tunnel: [w1489] -> w170
            tunnel: [w1487] -> w169
            tunnel: [w1489] -> w168
            tunnel: [w1488] -> w164
            tunnel: [w1487] -> w161
            tunnel: w157 -> [w1484]
            tunnel: [w1483] -> w155
            tunnel: w146 -> [w1482]
            tunnel: [w1482] -> w145
            tunnel: [w1481] -> w143
            tunnel: [w1480] -> w134
            tunnel: w345 -> [w1783]
            tunnel: [w1780] -> w319
            tunnel: w344 -> [w1796]
            tunnel: [w1796] -> w318
            tunnel: w343 -> [w1795]
            tunnel: [w1795] -> w317
            tunnel: w342 -> [w1794]
            tunnel: [w1794] -> w316
            tunnel: w341 -> [w1793]
            tunnel: [w1793] -> w315
            tunnel: w340 -> [w1792]
            tunnel: [w1792] -> w314
            tunnel: w339 -> [w1791]
            tunnel: [w1791] -> w313
            tunnel: [w1784] -> w312
            tunnel: w338 -> [w1777]
            tunnel: w337 -> [w1785]
            tunnel: w336 -> [w1784]
            tunnel: w335 -> [w1786]
            tunnel: [w1783] -> w311
            tunnel: w328 -> [w1782]
            tunnel: w325 -> [w1781]
            tunnel: [w1779] -> w310
            tunnel: [w1767] -> w309
            tunnel: w306 -> [w1778]
            tunnel: w301 -> [w1775]
            tunnel: w300 -> [w1774]
            tunnel: [w1776] -> w297
            tunnel: [w1773] -> w294
            tunnel: [w1772] -> w291
            tunnel: [w1768] -> w290
            tunnel: [w1766] -> w262
            tunnel: w261 -> [w1766]
            tunnel: w236 -> [w1765]
            tunnel: w235 -> [w1764]
            tunnel: w234 -> [w1763]
            tunnel: w233 -> [w1761]
            tunnel: [w1759] -> w232
            tunnel: [w1758] -> w231
            tunnel: [w1757] -> w230
            tunnel: [w1756] -> w229
            tunnel: w218 -> [w1760]
            tunnel: w214 -> [w1762]
            tunnel: [w1759] -> w210
            tunnel: [w1758] -> w209
            tunnel: [w1757] -> w208
            tunnel: [w1756] -> w207
            tunnel: [w1755] -> w190
            tunnel: w189 -> [w1755]
            tunnel: [w1754] -> w187
            tunnel: w186 -> [w1754]
            tunnel: w170 -> [w1753]
            tunnel: w169 -> [w1752]
            tunnel: w168 -> [w1751]
            tunnel: [w1751] -> w167
            tunnel: [w1750] -> w165
            tunnel: w164 -> [w1750]
            tunnel: w161 -> [w1749]
            tunnel: [w1749] -> w160
            tunnel: w155 -> [w1748]
            tunnel: [w1746] -> w154
            tunnel: w145 -> [w1745]
            tunnel: [w1744] -> w144
            tunnel: w143 -> [w1744]
            tunnel: [w1743] -> w135
            tunnel: w134 -> [w1743]
            tunnel: w319 -> [w1834]
            tunnel: [w1841] -> w359
            tunnel: [w1840] -> w358
            tunnel: w318 -> [w1840]
            tunnel: [w1835] -> w355
            tunnel: w317 -> [w1835]
            tunnel: [w1839] -> w353
            tunnel: w316 -> [w1839]
            tunnel: [w1838] -> w351
            tunnel: w315 -> [w1838]
            tunnel: [w1837] -> w349
            tunnel: w314 -> [w1837]
            tunnel: [w1836] -> w347
            tunnel: w313 -> [w1836]
            tunnel: w312 -> [w1823]
            tunnel: w311 -> [w1824]
            tunnel: w310 -> [w1802]
            tunnel: [w1802] -> w322
            tunnel: w309 -> [w1825]
            tunnel: [w1825] -> w320
            tunnel: [w1827] -> w298
            tunnel: w297 -> [w1827]
            tunnel: [w1828] -> w295
            tunnel: w294 -> [w1828]
            tunnel: [w1829] -> w292
            tunnel: w291 -> [w1829]
            tunnel: w290 -> [w1833]
            tunnel: [w1822] -> w263
            tunnel: w262 -> [w1822]
            tunnel: w232 -> [w1819]
            tunnel: w231 -> [w1818]
            tunnel: w230 -> [w1817]
            tunnel: w229 -> [w1816]
            tunnel: w210 -> [w1815]
            tunnel: w209 -> [w1814]
            tunnel: w208 -> [w1813]
            tunnel: w207 -> [w1812]
            tunnel: [w1815] -> w205
            tunnel: [w1814] -> w203
            tunnel: [w1813] -> w201
            tunnel: [w1812] -> w199
            tunnel: w190 -> [w1811]
            tunnel: [w1810] -> w188
            tunnel: w187 -> [w1810]
            tunnel: w167 -> [w1807]
            tunnel: [w1806] -> w166
            tunnel: w165 -> [w1806]
            tunnel: w160 -> [w1805]
            tunnel: w154 -> [w1803]
            tunnel: [w1803] -> w151
            tunnel: w144 -> [w1801]
            tunnel: [w1801] -> w140
            tunnel: [w1800] -> w136
            tunnel: w135 -> [w1800]
            tunnel: w359 -> [w1857]
            tunnel: w358 -> [w1872]
            tunnel: w355 -> [w1866]
            tunnel: w353 -> [w1871]
            tunnel: w351 -> [w1868]
            tunnel: w349 -> [w1870]
            tunnel: w347 -> [w1869]
            tunnel: w322 -> [w1862]
            tunnel: w320 -> [w1861]
            tunnel: w298 -> [w1860]
            tunnel: w295 -> [w1859]
            tunnel: w292 -> [w1858]
            tunnel: [w1851] -> w183
            tunnel: [w1872] -> w275
            tunnel: [w1866] -> w274
            tunnel: [w1871] -> w273
            tunnel: [w1868] -> w272
            tunnel: [w1870] -> w271
            tunnel: [w1869] -> w270
            tunnel: [w1862] -> w269
            tunnel: [w1861] -> w268
            tunnel: [w1860] -> w267
            tunnel: [w1859] -> w266
            tunnel: [w1858] -> w265
            tunnel: [w1856] -> w264
            tunnel: w263 -> [w1856]
            tunnel: [w1855] -> w206
            tunnel: w205 -> [w1855]
            tunnel: [w1854] -> w204
            tunnel: w203 -> [w1854]
            tunnel: [w1853] -> w202
            tunnel: w201 -> [w1853]
            tunnel: [w1852] -> w200
            tunnel: w199 -> [w1852]
            tunnel: w188 -> [w1850]
            tunnel: [w1849] -> w173
            tunnel: [w1848] -> w172
            tunnel: w166 -> [w1847]
            tunnel: [w1846] -> w163
            tunnel: [w1845] -> w162
            tunnel: [w1844] -> w152
            tunnel: w151 -> [w1844]
            tunnel: [w1843] -> w141
            tunnel: w140 -> [w1843]
            tunnel: [w1842] -> w137
            tunnel: w136 -> [w1842]
            tunnel: w275 -> [w1922]
            tunnel: w274 -> [w1921]
            tunnel: w273 -> [w1920]
            tunnel: w272 -> [w1919]
            tunnel: w271 -> [w1918]
            tunnel: w270 -> [w1917]
            tunnel: w269 -> [w1916]
            tunnel: w268 -> [w1915]
            tunnel: w267 -> [w1914]
            tunnel: w266 -> [w1913]
            tunnel: w265 -> [w1912]
            tunnel: w264 -> [w1905]
            tunnel: [w1922] -> w257
            tunnel: [w1921] -> w256
            tunnel: [w1920] -> w255
            tunnel: [w1919] -> w254
            tunnel: [w1918] -> w253
            tunnel: [w1917] -> w252
            tunnel: [w1916] -> w251
            tunnel: [w1915] -> w250
            tunnel: [w1914] -> w249
            tunnel: [w1913] -> w248
            tunnel: [w1912] -> w247
            tunnel: [w1905] -> w246
            tunnel: [w1904] -> w245
            tunnel: w206 -> [w1902]
            tunnel: w204 -> [w1901]
            tunnel: w202 -> [w1900]
            tunnel: w200 -> [w1899]
            tunnel: [w1902] -> w198
            tunnel: [w1901] -> w196
            tunnel: [w1900] -> w194
            tunnel: [w1899] -> w192
            tunnel: w173 -> [w1898]
            tunnel: w172 -> [w1897]
            tunnel: [w1892] -> w171
            tunnel: w163 -> [w1891]
            tunnel: w162 -> [w1890]
            tunnel: [w1889] -> w153
            tunnel: w152 -> [w1889]
            tunnel: [w1888] -> w142
            tunnel: w141 -> [w1888]
            tunnel: [w1887] -> w138
            tunnel: w137 -> [w1887]
            tunnel: [w1936] -> w293
            tunnel: [w1937] -> w296
            tunnel: [w1938] -> w299
            tunnel: [w1939] -> w321
            tunnel: [w1940] -> w323
            tunnel: [w1941] -> w348
            tunnel: [w1942] -> w350
            tunnel: [w1943] -> w352
            tunnel: [w1944] -> w354
            tunnel: [w1945] -> w356
            tunnel: [w1946] -> w357
            tunnel: w257 -> [w1946]
            tunnel: w256 -> [w1945]
            tunnel: w255 -> [w1944]
            tunnel: w254 -> [w1943]
            tunnel: w253 -> [w1942]
            tunnel: w252 -> [w1941]
            tunnel: w251 -> [w1940]
            tunnel: w250 -> [w1939]
            tunnel: w249 -> [w1938]
            tunnel: w248 -> [w1937]
            tunnel: w247 -> [w1936]
            tunnel: w246 -> [w1932]
            tunnel: w245 -> [w1931]
            tunnel: [w1930] -> w197
            tunnel: w198 -> [w1930]
            tunnel: [w1929] -> w195
            tunnel: w196 -> [w1929]
            tunnel: [w1928] -> w193
            tunnel: w194 -> [w1928]
            tunnel: [w1927] -> w191
            tunnel: w192 -> [w1927]
            tunnel: [w1926] -> w185
            tunnel: w171 -> [w1926]
            tunnel: [w1925] -> w150
            tunnel: w153 -> [w1925]
            tunnel: w142 -> [w1924]
            tunnel: [w1924] -> w139
            tunnel: w138 -> [w1923]
            tunnel: [w1923] -> w133
            frame #0 {
              n18 = Tick Count (ms)() -> (millisecond timer value=w389:u32)
            }
            frame #1 {
              n19 = while {
                tunnel: w426 -> [w436]
                tunnel: [w435] -> w425
                tunnel: [w431] -> w424
                tunnel: w412 -> [w433]
                tunnel: w402 -> [w432]
                tunnel: [w430] -> w404
                tunnel: [w429] -> w403
                stop <- w437 stop-if-true
                n20 = event shown="[15] \"Get Values\": Value Change" {
                  selector: _ -> [_ _ _ _ _ _ _ _ _ _ _ _ _ _ _ _ _ _ _ _ _]
                  dyn-events: _ -> [_ _ _ _ _ _ _ _ _ _ _ _ _ _ _ _ _ _ _ _ _]
                  timeout: 1 -> [_ _ _ _ _ _ _ _ _ _ _ _ _ _ _ _ _ _ _ _ _]
                  tunnel: [TRUE ("Set Gauge to Zero") w451 w502 w553 w578 w602 w631 w660 w699 w737 w795 w854 w908 w962 w1044 w1126 w1200 w1274 w1348 "Set Gauge to Zero" _] -> w437
                  tunnel: w436 -> [w444 w450 w497 w550 w572 w600 w628 w656 w694 w736 w790 w850 w906 w960 w1042 w1124 w1196 w1272 w1346 w1426 w1451]
                  tunnel: [w443 w449 w496 w549 w571 w599 w625 w658 w693 w734 w792 w852 w905 w959 w1041 w1123 w1198 w1271 w1345 w1425 w1450] -> w435
                  tunnel: [w442 w448 w495 w548 w570 w598 w624 w657 w692 w735 w791 w851 w904 w958 w1040 w1122 w1197 w1270 w1344 w1424 w1449] -> w431
                  tunnel: w433 -> [_ _ _ _ _ _ _ _ _ _ _ _ _ _ _ _ _ _ _ w1422 _]
                  tunnel: w432 -> [w440 w447 w500 w547 w575 w597 w629 w653 w697 w733 w789 w849 w903 w957 w1037 w1121 w1195 w1269 w1343 w1417 w1443]
                  tunnel: [w438 w446 w499 w546 w574 w596 w627 w655 w696 w732 w794 w848 w902 w956 w1039 w1120 w1194 w1268 w1342 w1416 w1442] -> w430
                  tunnel: [w439 w445 w498 w545 w573 w595 w626 w654 w695 w731 w793 w847 w901 w955 w1038 w1119 w1193 w1267 w1341 w1415 w1441] -> w429
                  event Timeout {
                    n21 = event-data() -> ()  [unwired: 1 in, 1 out]
                    n22 = Unbundle(w444) -> ("VISA resource name out"=w443:refnum<visa-resource-name>, "error out"=w442:errorcluster)  [unwired: 2 out]
                    n23 = Unbundle(w440) -> ("VISA resource name out"=w438:refnum<visa-resource-name>, "error out"=w439:errorcluster)  [unwired: 2 out]
                  }
                  event "Setpoint\n START": Value Change {
                    n24 = event-data() -> ()  [unwired: 1 in, 1 out]
                    n25 = stacked-sequence {
                      tunnel: w450 -> [_ w457 _]
                      tunnel: [_ w456 _] -> w448
                      tunnel: [_ w455 _] -> w449
                      frame #0 {
                        n26 = property on="Setpoint\n START" class="Bool"("Blinking"=TRUE) -> ()  [unwired: 2 in, 2 out]
                        n27 = property on="ON" class="Bool (strict)"("Blinking"=FALSE) -> ()  [unwired: 2 in, 2 out]
                      }
                      frame #1 {
                        n28 = for {
                          N: 2 -> [_]
                          tunnel: w457 -> [w461]
                          tunnel: [w460] -> w456
                          tunnel: [w459] -> w455
                          i -> [w463]
                          n29 = flat-sequence {
                            tunnel: [w466] -> w462
                            tunnel: w463 -> [w465]
                            tunnel: [w484] -> w464
                            tunnel: w462 -> [w483]
                            tunnel: w461 -> [w485]
                            tunnel: [w482] -> w460
                            tunnel: [w481] -> w459
                            tunnel: w464 -> [w491]
                            tunnel: w463 -> [w490]
                            frame #0 {
                              n30 = case shown="0, Default" w465 {
                                tunnel: [w475 w477] -> w466
                                frame 0, Default {
                                n31 = Multiply(x=10.0, y="SP 1 input (°C)") -> (x*y=w472:dbl)
                                n32 = local read "RAM"() -> (w470:bool)
                                n33 = Number To Hexadecimal String(1:i16 5 ("width (-)"), 2:w472) -> (0:w474:string)
                                n34 = Select(t="*P012", s=w470, f="*P012") -> (s? t:f=w467:string)
                                n35 = Concatenate Strings(w467, w474) -> (w475:string)
                                }
                                frame 1 {
                                n36 = local read "RAM"() -> (w480:bool)
                                n37 = Select(t="*G01", s=w480, f="*R01") -> (s? t:f=w477:string)
                                }
                              }
                            }
                            frame #1 {
                              n38 = Unbundle(w485) -> ("VISA resource name out"=w486:refnum<visa-resource-name>, "error out"=w488:errorcluster, "Delay (ms)"=w487:u32, "Write/\nRead"=w489:bool)
                              n39 = call "I3252_Comm_Interface.vi"("VISA resource name in"=w486, "error in"=w488, "Delay (ms)"=w487, "Write"=w489, "String to Write"=w483, "Read"=w489) -> ("VISA resource name out"=w481:refnum<visa-resource-name>, "error out"=w482:errorcluster, "Read String"=w484:string)  [unwired: 2 in]
                            }
                            frame #2 {
                              n40 = case shown="0, Default" w490 {
                                tunnel: w491 -> [_ w493]
                                frame 0, Default {
                                }
                                frame 1 {
                                n41 = call "I3252_Edit_Setpoint.vi"("Read String"=w493) -> ("Setpoint is"=→"SP 1 is (°C)":dbl)
                                }
                              }
                            }
                          }
                        }
                      }
                      frame #2 {
                        n42 = property on="Setpoint\n START" class="Bool"("Blinking"=FALSE) -> ()  [unwired: 2 in, 2 out]
                      }
                    }
                    n43 = Unbundle(w447) -> ("VISA resource name out"=w446:refnum<visa-resource-name>, "error out"=w445:errorcluster)  [unwired: 2 out]
                    n44 = Not(x="Setpoint\n START") -> (.not. x?=w451:bool)
                  }
                  event "Setpoint\n START\n2": Value Change {
                    n45 = event-data() -> ()  [unwired: 1 in, 1 out]
                    n46 = stacked-sequence {
                      tunnel: w500 -> [_ w507 _]
                      tunnel: [_ w506 _] -> w498
                      tunnel: [_ w505 _] -> w499
                      frame #0 {
                        n47 = property on="Setpoint\n START\n2" class="Bool"("Blinking"=TRUE) -> ()  [unwired: 2 in, 2 out]
                        n48 = property on="ON 2" class="Bool (strict)"("Blinking"=FALSE) -> ()  [unwired: 2 in, 2 out]
                      }
                      frame #1 {
                        n49 = for {
                          N: 2 -> [_]
                          tunnel: w507 -> [w511]
                          tunnel: [w510] -> w506
                          tunnel: [w509] -> w505
                          i -> [w513]
                          n50 = flat-sequence {
                            tunnel: [w516] -> w512
                            tunnel: w513 -> [w515]
                            tunnel: [w534] -> w514
                            tunnel: w512 -> [w533]
                            tunnel: w511 -> [w535]
                            tunnel: [w532] -> w510
                            tunnel: [w531] -> w509
                            tunnel: w514 -> [w541]
                            tunnel: w513 -> [w540]
                            frame #0 {
                              n51 = case shown="0, Default" w515 {
                                tunnel: [w525 w527] -> w516
                                frame 0, Default {
                                n52 = Multiply(x=10.0, y="SP 2 input (°C)") -> (x*y=w523:dbl)
                                n53 = local read "RAM"() -> (w521:bool)
                                n54 = Number To Hexadecimal String(1:i16 5 ("width (-)"), 2:w523) -> (0:w524:string)
                                n55 = Select(t="*P012", s=w521, f="*P012") -> (s? t:f=w518:string)
                                n56 = Concatenate Strings(w518, w524) -> (w525:string)
                                }
                                frame 1 {
                                n57 = local read "RAM"() -> (w530:bool)
                                n58 = Select(t="*G01", s=w530, f="*R01") -> (s? t:f=w527:string)
                                }
                              }
                            }
                            frame #1 {
                              n59 = Unbundle(w535) -> ("VISA resource name out"=w536:refnum<visa-resource-name>, "error out"=w538:errorcluster, "Delay (ms) 2"=w537:u32, "Write/\nRead \n\n2"=w539:bool)
                              n60 = call "I3252_Comm_Interface.vi"("VISA resource name in"=w536, "error in"=w538, "Delay (ms)"=w537, "Write"=w539, "String to Write"=w533, "Read"=w539) -> ("VISA resource name out"=w531:refnum<visa-resource-name>, "error out"=w532:errorcluster, "Read String"=w534:string)  [unwired: 2 in]
                            }
                            frame #2 {
                              n61 = case shown="1" w540 {
                                tunnel: w541 -> [_ w543]
                                frame 0, Default {
                                }
                                frame 1 {
                                n62 = call "I3252_Edit_Setpoint.vi"("Read String"=w543) -> ("Setpoint is"=→"SP 2 is (°C)":dbl)
                                }
                              }
                            }
                          }
                        }
                      }
                      frame #2 {
                        n63 = property on="Setpoint\n START\n2" class="Bool"("Blinking"=FALSE) -> ()  [unwired: 2 in, 2 out]
                      }
                    }
                    n64 = Not(x="Setpoint\n START\n2") -> (.not. x?=w502:bool)
                    n65 = Unbundle(w497) -> ("VISA resource name out"=w496:refnum<visa-resource-name>, "error out"=w495:errorcluster)  [unwired: 2 out]
                  }
                  event "Standby": Value Change {
                    n66 = event-data() -> ()  [unwired: 1 in, 1 out]
                    n67 = flat-sequence {
                      tunnel: [w561] -> w551
                      tunnel: w551 -> [w565]
                      tunnel: w550 -> [w564]
                      tunnel: [w563] -> w548
                      tunnel: [w562] -> w549
                      frame #0 {
                        n68 = local read "Standby"() -> (w554:bool)
                        n69 = Select(t=TRUE, s=w554, f=FALSE) -> (s? t:f=w557:bool)
                        n70 = property on="Standby" class="Bool (strict)"("Blinking"=w557) -> ()  [unwired: 2 in, 2 out]
                      }
                      frame #1 {
                        n71 = local read "Standby"() -> (w559:bool)
                        n72 = Select(t="*D03", s=w559, f="*E03") -> (s? t:f=w561:string)
                      }
                      frame #2 {
                        n73 = Unbundle(w564) -> ("VISA resource name out"=w566:refnum<visa-resource-name>, "error out"=w568:errorcluster, "Delay (ms)"=w567:u32, "Write/\nRead"=w569:bool)
                        n74 = call "I3252_Comm_Interface.vi"("VISA resource name in"=w566, "error in"=w568, "Delay (ms)"=w567, "Write"=w569, "String to Write"=w565, "Read"=w569) -> ("VISA resource name out"=w562:refnum<visa-resource-name>, "error out"=w563:errorcluster)  [unwired: 2 in, 1 out]
                      }
                    }
                    n75 = Not(x="Standby") -> (.not. x?=w553:bool)
                    n76 = Unbundle(w547) -> ("VISA resource name out"=w546:refnum<visa-resource-name>, "error out"=w545:errorcluster)  [unwired: 2 out]
                  }
                  event "Standby\n2": Value Change {
                    n77 = event-data() -> ()  [unwired: 1 in, 1 out]
                    n78 = flat-sequence {
                      tunnel: [w586] -> w577
                      tunnel: w577 -> [w590]
                      tunnel: w575 -> [w589]
                      tunnel: [w588] -> w573
                      tunnel: [w587] -> w574
                      frame #0 {
                        n79 = local read "Standby\n2"() -> (w580:bool)
                        n80 = Select(t=TRUE, s=w580, f=FALSE) -> (s? t:f=w579:bool)
                        n81 = property on="Standby\n2" class="Bool (strict)"("Blinking"=w579) -> ()  [unwired: 2 in, 2 out]
                      }
                      frame #1 {
                        n82 = local read "Standby\n2"() -> (w584:bool)
                        n83 = Select(t="*D03", s=w584, f="*E03") -> (s? t:f=w586:string)
                      }
                      frame #2 {
                        n84 = Unbundle(w589) -> ("VISA resource name out"=w591:refnum<visa-resource-name>, "error out"=w593:errorcluster, "Delay (ms) 2"=w592:u32, "Write/\nRead \n\n2"=w594:bool)
                        n85 = call "I3252_Comm_Interface.vi"("VISA resource name in"=w591, "error in"=w593, "Delay (ms)"=w592, "Write"=w594, "String to Write"=w590, "Read"=w594) -> ("VISA resource name out"=w587:refnum<visa-resource-name>, "error out"=w588:errorcluster)  [unwired: 2 in, 1 out]
                      }
                    }
                    n86 = Not(x="Standby\n2") -> (.not. x?=w578:bool)
                    n87 = Unbundle(w572) -> ("VISA resource name out"=w571:refnum<visa-resource-name>, "error out"=w570:errorcluster)  [unwired: 2 out]
                  }
                  event "Set Command": Value Change {
                    n88 = event-data() -> ()  [unwired: 1 in, 1 out]
                    n89 = stacked-sequence {
                      tunnel: w600 -> [_ w607 _]
                      tunnel: [_ w606 _] -> w599
                      tunnel: [_ w605 _] -> w598
                      frame #0 {
                        n90 = property on="Set Command" class="Bool"("Blinking"=TRUE) -> ()  [unwired: 2 in, 2 out]
                        n91 = property on="ON" class="Bool (strict)"("Blinking"=FALSE) -> ()  [unwired: 2 in, 2 out]
                      }
                      frame #1 {
                        n92 = flat-sequence {
                          tunnel: [w612] -> w609
                          tunnel: [w615] -> w608
                          tunnel: w609 -> [w616]
                          tunnel: w607 -> [w617]
                          tunnel: [w614] -> w606
                          tunnel: [w613] -> w605
                          tunnel: w608 -> [w622]
                          frame #0 {
                            n93 = Concatenate Strings("*", "Command input") -> (w612:string)
                          }
                          frame #1 {
                            n94 = Unbundle(w617) -> ("VISA resource name out"=w621:refnum<visa-resource-name>, "error out"=w619:errorcluster, "Delay (ms)"=w620:u32, "Write/\nRead"=w618:bool)
                            n95 = call "I3252_Comm_Interface.vi"("VISA resource name in"=w621, "error in"=w619, "Delay (ms)"=w620, "Write"=w618, "String to Write"=w616, "Read"=w618) -> ("VISA resource name out"=w614:refnum<visa-resource-name>, "error out"=w613:errorcluster, "Read String"=w615:string)  [unwired: 2 in]
                          }
                          frame #2 {
                            "Command output" <- w622
                          }
                        }
                      }
                      frame #2 {
                        n96 = property on="Set Command" class="Bool"("Blinking"=FALSE) -> ()  [unwired: 2 in, 2 out]
                      }
                    }
                    n97 = Not(x="Set Command") -> (.not. x?=w602:bool)
                    n98 = Unbundle(w597) -> ("VISA resource name out"=w596:refnum<visa-resource-name>, "error out"=w595:errorcluster)  [unwired: 2 out]
                  }
                  event "Set Command\n\n 2": Value Change {
                    n99 = event-data() -> ()  [unwired: 1 in, 1 out]
                    n100 = stacked-sequence {
                      tunnel: w629 -> [_ w636 _]
                      tunnel: [_ w635 _] -> w627
                      tunnel: [_ w634 _] -> w626
                      frame #0 {
                        n101 = property on="Set Command\n\n 2" class="Bool"("Blinking"=TRUE) -> ()  [unwired: 2 in, 2 out]
                        n102 = property on="ON 2" class="Bool (strict)"("Blinking"=FALSE) -> ()  [unwired: 2 in, 2 out]
                      }
                      frame #1 {
                        n103 = flat-sequence {
                          tunnel: [w641] -> w638
                          tunnel: [w644] -> w637
                          tunnel: w638 -> [w645]
                          tunnel: w636 -> [w646]
                          tunnel: [w643] -> w635
                          tunnel: [w642] -> w634
                          tunnel: w637 -> [w651]
                          frame #0 {
                            n104 = Concatenate Strings("*", "Command input 2") -> (w641:string)
                          }
                          frame #1 {
                            n105 = Unbundle(w646) -> ("VISA resource name out"=w650:refnum<visa-resource-name>, "error out"=w648:errorcluster, "Delay (ms) 2"=w649:u32, "Write/\nRead \n\n2"=w647:bool)
                            n106 = call "I3252_Comm_Interface.vi"("VISA resource name in"=w650, "error in"=w648, "Delay (ms)"=w649, "Write"=w647, "String to Write"=w645, "Read"=w647) -> ("VISA resource name out"=w643:refnum<visa-resource-name>, "error out"=w642:errorcluster, "Read String"=w644:string)  [unwired: 2 in]
                          }
                          frame #2 {
                            "Command output 2" <- w651
                          }
                        }
                      }
                      frame #2 {
                        n107 = property on="Set Command\n\n 2" class="Bool"("Blinking"=FALSE) -> ()  [unwired: 2 in, 2 out]
                      }
                    }
                    n108 = Not(x="Set Command\n\n 2") -> (.not. x?=w631:bool)
                    n109 = Unbundle(w628) -> ("VISA resource name out"=w625:refnum<visa-resource-name>, "error out"=w624:errorcluster)  [unwired: 2 out]
                  }
                  event "Reset\nSTOP": Value Change {
                    n110 = event-data() -> ()  [unwired: 1 in, 1 out]
                    n111 = stacked-sequence {
                      tunnel: [_ w667 _] -> w657
                      tunnel: [_ w666 _] -> w658
                      tunnel: w656 -> [_ w664 _]
                      frame #0 {
                        n112 = property on="Reset\nSTOP" class="Bool"("Blinking"=TRUE) -> ()  [unwired: 2 in, 2 out]
                        n113 = property on="ON" class="Bool (strict)"("Blinking"=FALSE) -> ()  [unwired: 2 in, 2 out]
                      }
                      frame #1 {
                        n114 = for {
                          N: 2 -> [_]
                          tunnel: [w673] -> w667
                          tunnel: [w672] -> w666
                          tunnel: w664 -> [w671]
                          i -> [w669]
                          n115 = flat-sequence {
                            tunnel: w669 -> [w675]
                            tunnel: [w674] -> w670
                            tunnel: [w680] -> w673
                            tunnel: [w681] -> w672
                            tunnel: w671 -> [w682]
                            tunnel: w670 -> [w679]
                            tunnel: [w678] -> w668
                            tunnel: w669 -> [w688]
                            tunnel: w668 -> [w687]
                            frame #0 {
                              n116 = case shown="0, Default" w675 {
                                tunnel: ["*Z02" "*G01"] -> w674
                                frame 0, Default {
                                }
                                frame 1 {
                                }
                              }
                            }
                            frame #1 {
                              n117 = Unbundle(w682) -> ("VISA resource name out"=w683:refnum<visa-resource-name>, "error out"=w685:errorcluster, "Delay (ms)"=w684:u32, "Write/\nRead"=w686:bool)
                              n118 = call "I3252_Comm_Interface.vi"("VISA resource name in"=w683, "error in"=w685, "Delay (ms)"=w684, "Write"=w686, "String to Write"=w679, "Read"=w686) -> ("VISA resource name out"=w681:refnum<visa-resource-name>, "error out"=w680:errorcluster, "Read String"=w678:string)  [unwired: 2 in]
                            }
                            frame #2 {
                              n119 = case shown="0, Default" w688 {
                                tunnel: w687 -> [_ w690]
                                frame 0, Default {
                                }
                                frame 1 {
                                n120 = call "I3252_Edit_Setpoint.vi"("Read String"=w690) -> ("Setpoint is"=w689:dbl)
                                n121 = local write "SP 1 is (°C)"(w689) -> ()
                                }
                              }
                            }
                          }
                        }
                        n122 = Wait (ms)(milliseconds to wait=u32 4000) -> ()  [unwired: 1 out]
                      }
                      frame #2 {
                        n123 = property on="Reset\nSTOP" class="Bool"("Blinking"=FALSE) -> ()  [unwired: 2 in, 2 out]
                      }
                    }
                    n124 = Not(x="Reset\nSTOP") -> (.not. x?=w660:bool)
                    n125 = Unbundle(w653) -> ("VISA resource name out"=w655:refnum<visa-resource-name>, "error out"=w654:errorcluster)  [unwired: 2 out]
                  }
                  event "Reset\nSTOP 2": Value Change {
                    n126 = event-data() -> ()  [unwired: 1 in, 1 out]
                    n127 = stacked-sequence {
                      tunnel: [_ w706 _] -> w695
                      tunnel: [_ w705 _] -> w696
                      tunnel: w697 -> [_ w703 _]
                      frame #0 {
                        n128 = property on="Reset\nSTOP 2" class="Bool"("Blinking"=TRUE) -> ()  [unwired: 2 in, 2 out]
                        n129 = property on="ON 2" class="Bool (strict)"("Blinking"=FALSE) -> ()  [unwired: 2 in, 2 out]
                      }
                      frame #1 {
                        n130 = for {
                          N: 2 -> [_]
                          tunnel: [w712] -> w706
                          tunnel: [w711] -> w705
                          tunnel: w703 -> [w710]
                          i -> [w708]
                          n131 = flat-sequence {
                            tunnel: w708 -> [w714]
                            tunnel: [w713] -> w709
                            tunnel: [w719] -> w712
                            tunnel: [w720] -> w711
                            tunnel: w710 -> [w721]
                            tunnel: w709 -> [w718]
                            tunnel: [w717] -> w707
                            tunnel: w708 -> [w727]
                            tunnel: w707 -> [w726]
                            frame #0 {
                              n132 = case shown="0, Default" w714 {
                                tunnel: ["*Z02" "*G01"] -> w713
                                frame 0, Default {
                                }
                                frame 1 {
                                }
                              }
                            }
                            frame #1 {
                              n133 = Unbundle(w721) -> ("VISA resource name out"=w722:refnum<visa-resource-name>, "error out"=w724:errorcluster, "Delay (ms) 2"=w723:u32, "Write/\nRead \n\n2"=w725:bool)
                              n134 = call "I3252_Comm_Interface.vi"("VISA resource name in"=w722, "error in"=w724, "Delay (ms)"=w723, "Write"=w725, "String to Write"=w718, "Read"=w725) -> ("VISA resource name out"=w720:refnum<visa-resource-name>, "error out"=w719:errorcluster, "Read String"=w717:string)  [unwired: 2 in]
                            }
                            frame #2 {
                              n135 = case shown="1" w727 {
                                tunnel: w726 -> [_ w729]
                                frame 0, Default {
                                }
                                frame 1 {
                                n136 = call "I3252_Edit_Setpoint.vi"("Read String"=w729) -> ("Setpoint is"=w728:dbl)
                                n137 = local write "SP 2 is (°C)"(w728) -> ()
                                }
                              }
                            }
                          }
                        }
                        n138 = Wait (ms)(milliseconds to wait=u32 4000) -> ()  [unwired: 1 out]
                      }
                      frame #2 {
                        n139 = property on="Reset\nSTOP 2" class="Bool"("Blinking"=FALSE) -> ()  [unwired: 2 in, 2 out]
                      }
                    }
                    n140 = Not(x="Reset\nSTOP 2") -> (.not. x?=w699:bool)
                    n141 = Unbundle(w694) -> ("VISA resource name out"=w693:refnum<visa-resource-name>, "error out"=w692:errorcluster)  [unwired: 2 out]
                  }
                  event "Auto Tune": Value Change {
                    n142 = event-data() -> ()  [unwired: 1 in, 1 out]
                    n143 = stacked-sequence {
                      tunnel: w736 -> [_ w743 w788]
                      tunnel: [_ w742 _] -> w735
                      tunnel: [_ w741 _] -> w734
                      frame #0 {
                        n144 = property on="Auto Tune" class="Bool"("Blinking"=TRUE) -> ()  [unwired: 2 in, 2 out]
                        n145 = property on="ON" class="Bool (strict)"("Blinking"=FALSE) -> ()  [unwired: 2 in, 2 out]
                      }
                      frame #1 {
                        n146 = for {
                          N: 4 -> [_]
                          tunnel: [w748] -> w741
                          tunnel: [w747] -> w742
                          tunnel: w743 -> [w746]
                          i -> [w751]
                          n147 = flat-sequence {
                            tunnel: w751 -> [w753]
                            tunnel: [w752] -> w749
                            tunnel: w749 -> [w768]
                            tunnel: [w767] -> w750
                            tunnel: [w770] -> w748
                            tunnel: [w769] -> w747
                            tunnel: w746 -> [w766]
                            tunnel: w751 -> [w776]
                            tunnel: w750 -> [w775]
                            frame #0 {
                              n148 = case shown="0, Default" w753 {
                                tunnel: ["*V01" w756 "*W0C35" "*Z02"] -> w752
                                frame 0, Default {
                                }
                                frame 1 {
                                n149 = local read "(°C)"() -> (w755:dbl)
                                n150 = Add(x=20.0, y=w755) -> (x+y=w762:dbl)
                                n151 = Multiply(x=10.0, y=w762) -> (x*y=w759:dbl)
                                n152 = Number To Hexadecimal String(1:i16 5 ("width (-)"), 2:w759) -> (0:w758:string)
                                n153 = Concatenate Strings("*W012", w758) -> (w756:string)
                                }
                                frame 2 {
                                # "35 hex = \n00110101 bin"
                                }
                                frame 3 {
                                }
                              }
                            }
                            frame #1 {
                              n154 = Unbundle(w766) -> ("VISA resource name out"=w774:refnum<visa-resource-name>, "error out"=w772:errorcluster, "Delay (ms)"=w773:u32, "Write/\nRead"=w771:bool)
                              n155 = call "I3252_Comm_Interface.vi"("VISA resource name in"=w774, "error in"=w772, "Delay (ms)"=w773, "Write"=w771, "String to Write"=w768, "Read"=w771) -> ("VISA resource name out"=w770:refnum<visa-resource-name>, "error out"=w769:errorcluster, "Read String"=w767:string)  [unwired: 2 in]
                            }
                            frame #2 {
                              n156 = case shown="0, Default" w776 {
                                tunnel: w775 -> [w778]
                                frame 0, Default {
                                n157 = call <vilib>:"Space Constant.vi"() -> ("String"=w781:string)
                                n158 = Search/Split String(string=w778, search string/char (-)=w781) -> (match + rest of string=w780:string)  [unwired: 1 in, 2 out]
                                n159 = Fract/Exp String To Number(use system decimal point (T)=FALSE, string=w780) -> (number=w777:dbl)  [unwired: 2 in, 1 out]
                                n160 = local write "(°C)"(w777) -> ()
                                }
                              }
                            }
                          }
                        }
                        n161 = Wait (ms)(milliseconds to wait=u32 45000) -> ()  [unwired: 1 out]
                      }
                      frame #2 {
                        n162 = Unbundle(w788) -> ("VISA resource name out"=w787:refnum<visa-resource-name>, "error out"=w785:errorcluster, "Delay (ms)"=w786:u32, "Write/\nRead"=w784:bool)
                        n163 = property on="Auto Tune" class="Bool"("Blinking"=FALSE) -> ()  [unwired: 2 in, 2 out]
                        n164 = call "I3252_Comm_Interface.vi"("VISA resource name in"=w787, "error in"=w785, "Delay (ms)"=w786, "Write"=w784, "String to Write"="*W01200000", "Read"=w784) -> ()  [unwired: 2 in, 3 out]
                      }
                    }
                    n165 = Not(x="Auto Tune") -> (.not. x?=w737:bool)
                    n166 = Unbundle(w733) -> ("VISA resource name out"=w732:refnum<visa-resource-name>, "error out"=w731:errorcluster)  [unwired: 2 out]
                  }
                  event "Auto Tune 2": Value Change {
                    n167 = event-data() -> ()  [unwired: 1 in, 1 out]
                    n168 = stacked-sequence {
                      tunnel: w789 -> [_ w801 w846]
                      tunnel: [_ w800 _] -> w793
                      tunnel: [_ w799 _] -> w794
                      frame #0 {
                        n169 = property on="Auto Tune 2" class="Bool"("Blinking"=TRUE) -> ()  [unwired: 2 in, 2 out]
                        n170 = property on="ON" class="Bool (strict)"("Blinking"=FALSE) -> ()  [unwired: 2 in, 2 out]
                      }
                      frame #1 {
                        n171 = for {
                          N: 4 -> [_]
                          tunnel: [w806] -> w799
                          tunnel: [w805] -> w800
                          tunnel: w801 -> [w804]
                          i -> [w809]
                          n172 = flat-sequence {
                            tunnel: w809 -> [w811]
                            tunnel: [w810] -> w807
                            tunnel: w807 -> [w826]
                            tunnel: [w825] -> w808
                            tunnel: [w828] -> w806
                            tunnel: [w827] -> w805
                            tunnel: w804 -> [w824]
                            tunnel: w809 -> [w834]
                            tunnel: w808 -> [w833]
                            frame #0 {
                              n173 = case shown="1" w811 {
                                tunnel: ["*V01" w814 "*W0C35" "*Z02"] -> w810
                                frame 0, Default {
                                }
                                frame 1 {
                                n174 = local read "(°C) 2"() -> (w813:dbl)
                                n175 = Add(x=20.0, y=w813) -> (x+y=w820:dbl)
                                n176 = Multiply(x=10.0, y=w820) -> (x*y=w817:dbl)
                                n177 = Number To Hexadecimal String(1:i16 5 ("width (-)"), 2:w817) -> (0:w816:string)
                                n178 = Concatenate Strings("*W012", w816) -> (w814:string)
                                }
                                frame 2 {
                                # "35 hex = \n00110101 bin"
                                }
                                frame 3 {
                                }
                              }
                            }
                            frame #1 {
                              n179 = Unbundle(w824) -> ("VISA resource name out"=w832:refnum<visa-resource-name>, "error out"=w830:errorcluster, "Delay (ms) 2"=w831:u32, "Write/\nRead \n\n2"=w829:bool)
                              n180 = call "I3252_Comm_Interface.vi"("VISA resource name in"=w832, "error in"=w830, "Delay (ms)"=w831, "Write"=w829, "String to Write"=w826, "Read"=w829) -> ("VISA resource name out"=w828:refnum<visa-resource-name>, "error out"=w827:errorcluster, "Read String"=w825:string)  [unwired: 2 in]
                            }
                            frame #2 {
                              n181 = case shown="0, Default" w834 {
                                tunnel: w833 -> [w836]
                                frame 0, Default {
                                n182 = call <vilib>:"Space Constant.vi"() -> ("String"=w839:string)
                                n183 = Search/Split String(string=w836, search string/char (-)=w839) -> (match + rest of string=w838:string)  [unwired: 1 in, 2 out]
                                n184 = Fract/Exp String To Number(use system decimal point (T)=FALSE, string=w838) -> (number=w835:dbl)  [unwired: 2 in, 1 out]
                                n185 = local write "(°C) 2"(w835) -> ()
                                }
                              }
                            }
                          }
                        }
                        n186 = Wait (ms)(milliseconds to wait=u32 45000) -> ()  [unwired: 1 out]
                      }
                      frame #2 {
                        n187 = Unbundle(w846) -> ("VISA resource name out"=w845:refnum<visa-resource-name>, "error out"=w843:errorcluster, "Delay (ms) 2"=w844:u32, "Write/\nRead \n\n2"=w842:bool)
                        n188 = property on="Auto Tune 2" class="Bool"("Blinking"=FALSE) -> ()  [unwired: 2 in, 2 out]
                        n189 = call "I3252_Comm_Interface.vi"("VISA resource name in"=w845, "error in"=w843, "Delay (ms)"=w844, "Write"=w842, "String to Write"="*W01200000", "Read"=w842) -> ()  [unwired: 2 in, 3 out]
                      }
                    }
                    n190 = Not(x="Auto Tune 2") -> (.not. x?=w795:bool)
                    n191 = Unbundle(w790) -> ("VISA resource name out"=w792:refnum<visa-resource-name>, "error out"=w791:errorcluster)  [unwired: 2 out]
                  }
                  event "Write LOW/HI": Value Change {
                    n192 = event-data() -> ()  [unwired: 1 in, 1 out]
                    n193 = stacked-sequence {
                      tunnel: [_ w859 _] -> w852
                      tunnel: [_ w858 _] -> w851
                      tunnel: w850 -> [_ w857 _]
                      frame #0 {
                        n194 = property on="Write LOW/HI" class="Bool"("Blinking"=TRUE) -> ()  [unwired: 2 in, 2 out]
                        n195 = property on="ON" class="Bool (strict)"("Blinking"=FALSE) -> ()  [unwired: 2 in, 2 out]
                      }
                      frame #1 {
                        n196 = for {
                          N: 4 -> [_]
                          tunnel: [w863] -> w859
                          tunnel: [w862] -> w858
                          tunnel: w857 -> [w861]
                          i -> [w865]
                          n197 = flat-sequence {
                            tunnel: w865 -> [w867]
                            tunnel: [w868] -> w864
                            tunnel: w864 -> [w882]
                            tunnel: [w883] -> w866
                            tunnel: [w885] -> w863
                            tunnel: [w884] -> w862
                            tunnel: w861 -> [w881]
                            tunnel: w866 -> [w891]
                            tunnel: w865 -> [w890]
                            frame #0 {
                              n198 = case shown="0, Default" w867 {
                                tunnel: [w870 w876 "*R27" "*R28"] -> w868
                                frame 0, Default {
                                n199 = Number To Hexadecimal String(1:i16 2 ("width (-)"), 2:"% LOW Sollwert") -> (0:w871:string)
                                n200 = Concatenate Strings("*W27", w871) -> (w870:string)
                                }
                                frame 1 {
                                n201 = Number To Hexadecimal String(1:i16 2 ("width (-)"), 2:"% High Sollwert") -> (0:w877:string)
                                n202 = Concatenate Strings("*W28", w877) -> (w876:string)
                                }
                                frame 2 {
                                }
                                frame 3 {
                                }
                              }
                            }
                            frame #1 {
                              n203 = Unbundle(w881) -> ("VISA resource name out"=w889:refnum<visa-resource-name>, "error out"=w887:errorcluster, "Delay (ms)"=w888:u32, "Write/\nRead"=w886:bool)
                              n204 = call "I3252_Comm_Interface.vi"("VISA resource name in"=w889, "error in"=w887, "Delay (ms)"=w888, "Write"=w886, "String to Write"=w882, "Read"=w886) -> ("VISA resource name out"=w885:refnum<visa-resource-name>, "error out"=w884:errorcluster, "Read String"=w883:string)  [unwired: 2 in]
                            }
                            frame #2 {
                              n205 = case shown="0, Default" w890 {
                                tunnel: w891 -> [_ w895 w899]
                                frame 0, Default {
                                }
                                frame 2 {
                                n206 = String Subset(string=w895, offset (0)=3) -> (substring=w893:string)  [unwired: 1 in]
                                n207 = Hexadecimal String To Number(string=w893) -> (number=→"% LOW Istwert":u32)  [unwired: 2 in, 1 out]
                                }
                                frame 3 {
                                n208 = String Subset(string=w899, offset (0)=3) -> (substring=w897:string)  [unwired: 1 in]
                                n209 = Hexadecimal String To Number(string=w897) -> (number=→"% HIGH Istwert":u32)  [unwired: 2 in, 1 out]
                                }
                              }
                            }
                          }
                        }
                      }
                      frame #2 {
                        n210 = property on="Write LOW/HI" class="Bool"("Blinking"=FALSE) -> ()  [unwired: 2 in, 2 out]
                      }
                    }
                    n211 = Not(x="Write LOW/HI") -> (.not. x?=w854:bool)
                    n212 = Unbundle(w849) -> ("VISA resource name out"=w848:refnum<visa-resource-name>, "error out"=w847:errorcluster)  [unwired: 2 out]
                  }
                  event "Write LOW/HI 2": Value Change {
                    n213 = event-data() -> ()  [unwired: 1 in, 1 out]
                    n214 = stacked-sequence {
                      tunnel: [_ w913 _] -> w902
                      tunnel: [_ w912 _] -> w901
                      tunnel: w903 -> [_ w911 _]
                      frame #0 {
                        n215 = property on="Write LOW/HI 2" class="Bool"("Blinking"=TRUE) -> ()  [unwired: 2 in, 2 out]
                        n216 = property on="ON 2" class="Bool (strict)"("Blinking"=FALSE) -> ()  [unwired: 2 in, 2 out]
                      }
                      frame #1 {
                        n217 = for {
                          N: 4 -> [_]
                          tunnel: [w917] -> w913
                          tunnel: [w916] -> w912
                          tunnel: w911 -> [w915]
                          i -> [w919]
                          n218 = flat-sequence {
                            tunnel: w919 -> [w921]
                            tunnel: [w922] -> w918
                            tunnel: w918 -> [w936]
                            tunnel: [w937] -> w920
                            tunnel: [w939] -> w917
                            tunnel: [w938] -> w916
                            tunnel: w915 -> [w935]
                            tunnel: w920 -> [w945]
                            tunnel: w919 -> [w944]
                            frame #0 {
                              n219 = case shown="0, Default" w921 {
                                tunnel: [w925 w930 "*R27" "*R28"] -> w922
                                frame 0, Default {
                                n220 = Number To Hexadecimal String(1:i16 2 ("width (-)"), 2:"% LOW Sollwert 2") -> (0:w926:string)
                                n221 = Concatenate Strings("*W27", w926) -> (w925:string)
                                }
                                frame 1 {
                                n222 = Number To Hexadecimal String(1:i16 2 ("width (-)"), 2:"% High Sollwert 2") -> (0:w931:string)
                                n223 = Concatenate Strings("*W28", w931) -> (w930:string)
                                }
                                frame 2 {
                                }
                                frame 3 {
                                }
                              }
                            }
                            frame #1 {
                              n224 = Unbundle(w935) -> ("VISA resource name out"=w943:refnum<visa-resource-name>, "error out"=w941:errorcluster, "Delay (ms) 2"=w942:u32, "Write/\nRead \n\n2"=w940:bool)
                              n225 = call "I3252_Comm_Interface.vi"("VISA resource name in"=w943, "error in"=w941, "Delay (ms)"=w942, "Write"=w940, "String to Write"=w936, "Read"=w940) -> ("VISA resource name out"=w939:refnum<visa-resource-name>, "error out"=w938:errorcluster, "Read String"=w937:string)  [unwired: 2 in]
                            }
                            frame #2 {
                              n226 = case shown="3" w944 {
                                tunnel: w945 -> [_ w949 w953]
                                frame 0, Default {
                                }
                                frame 2 {
                                n227 = String Subset(string=w949, offset (0)=3) -> (substring=w947:string)  [unwired: 1 in]
                                n228 = Hexadecimal String To Number(string=w947) -> (number=→"% LOW Istwert 2":u32)  [unwired: 2 in, 1 out]
                                }
                                frame 3 {
                                n229 = String Subset(string=w953, offset (0)=3) -> (substring=w951:string)  [unwired: 1 in]
                                n230 = Hexadecimal String To Number(string=w951) -> (number=→"% HIGH Istwert 2":u32)  [unwired: 2 in, 1 out]
                                }
                              }
                            }
                          }
                        }
                      }
                      frame #2 {
                        n231 = property on="Write LOW/HI 2" class="Bool"("Blinking"=FALSE) -> ()  [unwired: 2 in, 2 out]
                      }
                    }
                    n232 = Not(x="Write LOW/HI 2") -> (.not. x?=w908:bool)
                    n233 = Unbundle(w906) -> ("VISA resource name out"=w905:refnum<visa-resource-name>, "error out"=w904:errorcluster)  [unwired: 2 out]
                  }
                  event "Set PID": Value Change {
                    n234 = event-data() -> ()  [unwired: 1 in, 1 out]
                    n235 = stacked-sequence {
                      tunnel: w960 -> [_ w967 _]
                      tunnel: [_ w966 _] -> w959
                      tunnel: [_ w965 _] -> w958
                      frame #0 {
                        n236 = property on="Set PID" class="Bool"("Blinking"=TRUE) -> ()  [unwired: 2 in, 2 out]
                        n237 = property on="ON" class="Bool (strict)"("Blinking"=FALSE) -> ()  [unwired: 2 in, 2 out]
                      }
                      frame #1 {
                        n238 = for {
                          N: 6 -> [_]
                          tunnel: w967 -> [w971]
                          tunnel: [w970] -> w966
                          tunnel: [w969] -> w965
                          i -> [w973]
                          n239 = flat-sequence {
                            tunnel: w973 -> [w975]
                            tunnel: [w976] -> w972
                            tunnel: w972 -> [w1017]
                            tunnel: [w1013] -> w974
                            tunnel: w971 -> [w1016]
                            tunnel: [w1015] -> w969
                            tunnel: [w1014] -> w970
                            tunnel: w974 -> [w1023]
                            tunnel: w973 -> [w1022]
                            frame #0 {
                              n240 = case shown="2" w975 {
                                tunnel: [w983 w991 w999 w1001 w1005 w1009] -> w976
                                frame 0, Default {
                                n241 = local read "RAM"() -> (w977:bool)
                                n242 = Number To Hexadecimal String(1:i16 4 ("width (-)"), 2:"P (PB1) Sollwert") -> (0:w984:string)
                                n243 = Select(t="*P17", s=w977, f="*W17") -> (s? t:f=w978:string)
                                n244 = Concatenate Strings(w978, w984) -> (w983:string)
                                }
                                frame 1 {
                                n245 = local read "RAM"() -> (w985:bool)
                                n246 = Number To Hexadecimal String(1:i16 4 ("width (-)"), 2:"I ( Reset1) Sollwert") -> (0:w992:string)
                                n247 = Select(t="*P18", s=w985, f="*W18") -> (s? t:f=w987:string)
                                n248 = Concatenate Strings(w987, w992) -> (w991:string)
                                }
                                frame 2 {
                                n249 = local read "RAM"() -> (w994:bool)
                                n250 = Number To Hexadecimal String(1:i16 4 ("width (-)"), 2:"D (Rate) Sollwert") -> (0:w1000:string)
                                n251 = Select(t="*P19", s=w994, f="*W19") -> (s? t:f=w995:string)
                                n252 = Concatenate Strings(w995, w1000) -> (w999:string)
                                }
                                frame 3 {
                                n253 = local read "RAM"() -> (w1004:bool)
                                n254 = Select(t="*G17", s=w1004, f="*R17") -> (s? t:f=w1001:string)
                                }
                                frame 4 {
                                n255 = local read "RAM"() -> (w1008:bool)
                                n256 = Select(t="*G18", s=w1008, f="*R18") -> (s? t:f=w1005:string)
                                }
                                frame 5 {
                                n257 = local read "RAM"() -> (w1012:bool)
                                n258 = Select(t="*G19", s=w1012, f="*R19") -> (s? t:f=w1009:string)
                                }
                              }
                            }
                            frame #1 {
                              n259 = Unbundle(w1016) -> ("VISA resource name out"=w1021:refnum<visa-resource-name>, "error out"=w1019:errorcluster, "Delay (ms)"=w1020:u32, "Write/\nRead"=w1018:bool)
                              n260 = call "I3252_Comm_Interface.vi"("VISA resource name in"=w1021, "error in"=w1019, "Delay (ms)"=w1020, "Write"=w1018, "String to Write"=w1017, "Read"=w1018) -> ("VISA resource name out"=w1014:refnum<visa-resource-name>, "error out"=w1015:errorcluster, "Read String"=w1013:string)  [unwired: 2 in]
                            }
                            frame #2 {
                              n261 = case shown="4" w1022 {
                                tunnel: w1023 -> [_ w1027 w1031 w1035]
                                frame 0, Default {
                                }
                                frame 3 {
                                n262 = String Subset(string=w1027, offset (0)=3) -> (substring=w1025:string)  [unwired: 1 in]
                                n263 = Hexadecimal String To Number(string=w1025) -> (number=→"P (PB1) Istwert":u32)  [unwired: 2 in, 1 out]
                                }
                                frame 4 {
                                n264 = String Subset(string=w1031, offset (0)=3) -> (substring=w1029:string)  [unwired: 1 in]
                                n265 = Hexadecimal String To Number(string=w1029) -> (number=→"I ( Reset1) Istwert":u32)  [unwired: 2 in, 1 out]
                                }
                                frame 5 {
                                n266 = String Subset(string=w1035, offset (0)=3) -> (substring=w1033:string)  [unwired: 1 in]
                                n267 = Hexadecimal String To Number(string=w1033) -> (number=→"D (Rate) IstWert":u32)  [unwired: 2 in, 1 out]
                                }
                              }
                            }
                          }
                        }
                      }
                      frame #2 {
                        n268 = property on="Set PID" class="Bool"("Blinking"=FALSE) -> ()  [unwired: 2 in, 2 out]
                      }
                    }
                    n269 = Not(x="Set PID") -> (.not. x?=w962:bool)
                    n270 = Unbundle(w957) -> ("VISA resource name out"=w956:refnum<visa-resource-name>, "error out"=w955:errorcluster)  [unwired: 2 out]
                  }
                  event "Set PID 2": Value Change {
                    n271 = event-data() -> ()  [unwired: 1 in, 1 out]
                    n272 = stacked-sequence {
                      tunnel: w1037 -> [_ w1049 _]
                      tunnel: [_ w1048 _] -> w1039
                      tunnel: [_ w1047 _] -> w1038
                      frame #0 {
                        n273 = property on="Set PID 2" class="Bool"("Blinking"=TRUE) -> ()  [unwired: 2 in, 2 out]
                        n274 = property on="ON 2" class="Bool (strict)"("Blinking"=FALSE) -> ()  [unwired: 2 in, 2 out]
                      }
                      frame #1 {
                        n275 = for {
                          N: 6 -> [_]
                          tunnel: w1049 -> [w1053]
                          tunnel: [w1052] -> w1048
                          tunnel: [w1051] -> w1047
                          i -> [w1055]
                          n276 = flat-sequence {
                            tunnel: w1055 -> [w1057]
                            tunnel: [w1058] -> w1054
                            tunnel: w1054 -> [w1099]
                            tunnel: [w1095] -> w1056
                            tunnel: w1053 -> [w1098]
                            tunnel: [w1097] -> w1051
                            tunnel: [w1096] -> w1052
                            tunnel: w1056 -> [w1105]
                            tunnel: w1055 -> [w1104]
                            frame #0 {
                              n277 = case shown="0, Default" w1057 {
                                tunnel: [w1065 w1073 w1081 w1083 w1087 w1091] -> w1058
                                frame 0, Default {
                                n278 = local read "RAM 2"() -> (w1060:bool)
                                n279 = Number To Hexadecimal String(1:i16 4 ("width (-)"), 2:"P (PB1) Sollwert 2") -> (0:w1066:string)
                                n280 = Select(t="*P17", s=w1060, f="*W17") -> (s? t:f=w1061:string)
                                n281 = Concatenate Strings(w1061, w1066) -> (w1065:string)
                                }
                                frame 1 {
                                n282 = local read "RAM 2"() -> (w1068:bool)
                                n283 = Number To Hexadecimal String(1:i16 4 ("width (-)"), 2:"I ( Reset1) Sollwert 2") -> (0:w1074:string)
                                n284 = Select(t="*P18", s=w1068, f="*W18") -> (s? t:f=w1069:string)
                                n285 = Concatenate Strings(w1069, w1074) -> (w1073:string)
                                }
                                frame 2 {
                                n286 = local read "RAM 2"() -> (w1076:bool)
                                n287 = Number To Hexadecimal String(1:i16 4 ("width (-)"), 2:"D (Rate) Sollwert 2") -> (0:w1082:string)
                                n288 = Select(t="*P19", s=w1076, f="*W19") -> (s? t:f=w1077:string)
                                n289 = Concatenate Strings(w1077, w1082) -> (w1081:string)
                                }
                                frame 3 {
                                n290 = local read "RAM"() -> (w1086:bool)
                                n291 = Select(t="*G17", s=w1086, f="*R17") -> (s? t:f=w1083:string)
                                }
                                frame 4 {
                                n292 = local read "RAM"() -> (w1090:bool)
                                n293 = Select(t="*G18", s=w1090, f="*R18") -> (s? t:f=w1087:string)
                                }
                                frame 5 {
                                n294 = local read "RAM"() -> (w1094:bool)
                                n295 = Select(t="*G19", s=w1094, f="*R19") -> (s? t:f=w1091:string)
                                }
                              }
                            }
                            frame #1 {
                              n296 = Unbundle(w1098) -> ("VISA resource name out"=w1103:refnum<visa-resource-name>, "error out"=w1101:errorcluster, "Delay (ms) 2"=w1102:u32, "Write/\nRead \n\n2"=w1100:bool)
                              n297 = call "I3252_Comm_Interface.vi"("VISA resource name in"=w1103, "error in"=w1101, "Delay (ms)"=w1102, "Write"=w1100, "String to Write"=w1099, "Read"=w1100) -> ("VISA resource name out"=w1096:refnum<visa-resource-name>, "error out"=w1097:errorcluster, "Read String"=w1095:string)  [unwired: 2 in]
                            }
                            frame #2 {
                              n298 = case shown="0, Default" w1104 {
                                tunnel: w1105 -> [_ w1109 w1113 w1117]
                                frame 0, Default {
                                }
                                frame 3 {
                                n299 = String Subset(string=w1109, offset (0)=3) -> (substring=w1107:string)  [unwired: 1 in]
                                n300 = Hexadecimal String To Number(string=w1107) -> (number=→"P (PB1) Istwert 2":u32)  [unwired: 2 in, 1 out]
                                }
                                frame 4 {
                                n301 = String Subset(string=w1113, offset (0)=3) -> (substring=w1111:string)  [unwired: 1 in]
                                n302 = Hexadecimal String To Number(string=w1111) -> (number=→"I ( Reset1) Istwert 2":u32)  [unwired: 2 in, 1 out]
                                }
                                frame 5 {
                                n303 = String Subset(string=w1117, offset (0)=3) -> (substring=w1115:string)  [unwired: 1 in]
                                n304 = Hexadecimal String To Number(string=w1115) -> (number=→"D (Rate) IstWert 2":u32)  [unwired: 2 in, 1 out]
                                }
                              }
                            }
                          }
                        }
                      }
                      frame #2 {
                        n305 = property on="Set PID 2" class="Bool"("Blinking"=FALSE) -> ()  [unwired: 2 in, 2 out]
                      }
                    }
                    n306 = Not(x="Set PID 2") -> (.not. x?=w1044:bool)
                    n307 = Unbundle(w1042) -> ("VISA resource name out"=w1041:refnum<visa-resource-name>, "error out"=w1040:errorcluster)  [unwired: 2 out]
                  }
                  event "Get Values": Value Change {
                    n308 = event-data() -> ()  [unwired: 1 in, 1 out]
                    n309 = stacked-sequence {
                      tunnel: w1124 -> [_ w1131 _]
                      tunnel: [_ w1130 _] -> w1123
                      tunnel: [_ w1129 _] -> w1122
                      frame #0 {
                        n310 = property on="Get Values" class="Bool"("Blinking"=TRUE) -> ()  [unwired: 2 in, 2 out]
                        n311 = property on="ON" class="Bool (strict)"("Blinking"=FALSE) -> ()  [unwired: 2 in, 2 out]
                      }
                      frame #1 {
                        n312 = for {
                          N: 6 -> [_]
                          tunnel: w1131 -> [w1135]
                          tunnel: [w1134] -> w1130
                          tunnel: [w1133] -> w1129
                          i -> [w1137]
                          n313 = flat-sequence {
                            tunnel: w1137 -> [w1139]
                            tunnel: [w1140] -> w1136
                            tunnel: w1136 -> [w1162]
                            tunnel: [w1163] -> w1138
                            tunnel: w1135 -> [w1161]
                            tunnel: [w1160] -> w1133
                            tunnel: [w1159] -> w1134
                            tunnel: w1138 -> [w1169]
                            tunnel: w1137 -> [w1168]
                            frame #0 {
                              n314 = case shown="0, Default" w1139 {
                                tunnel: [w1143 w1147 w1151 "*R27" "*R28" w1157] -> w1140
                                frame 0, Default {
                                n315 = local read "RAM"() -> (w1144:bool)
                                n316 = Select(t="*G17", s=w1144, f="*R17") -> (s? t:f=w1143:string)
                                }
                                frame 1 {
                                n317 = local read "RAM"() -> (w1148:bool)
                                n318 = Select(t="*G18", s=w1148, f="*R18") -> (s? t:f=w1147:string)
                                }
                                frame 2 {
                                n319 = local read "RAM"() -> (w1152:bool)
                                n320 = Select(t="*G19", s=w1152, f="*R19") -> (s? t:f=w1151:string)
                                }
                                frame 3 {
                                }
                                frame 4 {
                                }
                                frame 5 {
                                n321 = local read "RAM"() -> (w1158:bool)
                                n322 = Select(t="*G01", s=w1158, f="*R01") -> (s? t:f=w1157:string)
                                }
                              }
                            }
                            frame #1 {
                              n323 = Unbundle(w1161) -> ("VISA resource name out"=w1167:refnum<visa-resource-name>, "error out"=w1165:errorcluster, "Delay (ms)"=w1166:u32, "Write/\nRead"=w1164:bool)
                              n324 = call "I3252_Comm_Interface.vi"("VISA resource name in"=w1167, "error in"=w1165, "Delay (ms)"=w1166, "Write"=w1164, "String to Write"=w1162, "Read"=w1164) -> ("VISA resource name out"=w1159:refnum<visa-resource-name>, "error out"=w1160:errorcluster, "Read String"=w1163:string)  [unwired: 2 in]
                            }
                            frame #2 {
                              n325 = case shown="1" w1168 {
                                tunnel: w1169 -> [w1171 w1175 w1179 w1183 w1187 w1191]
                                frame 0, Default {
                                n326 = String Subset(string=w1171, offset (0)=3) -> (substring=w1172:string)  [unwired: 1 in]
                                n327 = Hexadecimal String To Number(string=w1172) -> (number=w1170:u32)  [unwired: 2 in, 1 out]
                                n328 = local write "P (PB1) Sollwert"(w1170) -> ()
                                n329 = local write "P (PB1) Istwert"(w1170) -> ()
                                }
                                frame 1 {
                                n330 = String Subset(string=w1175, offset (0)=3) -> (substring=w1176:string)  [unwired: 1 in]
                                n331 = Hexadecimal String To Number(string=w1176) -> (number=w1174:u32)  [unwired: 2 in, 1 out]
                                n332 = local write "I ( Reset1) Sollwert"(w1174) -> ()
                                n333 = local write "I ( Reset1) Istwert"(w1174) -> ()
                                }
                                frame 2 {
                                n334 = String Subset(string=w1179, offset (0)=3) -> (substring=w1180:string)  [unwired: 1 in]
                                n335 = Hexadecimal String To Number(string=w1180) -> (number=w1178:u32)  [unwired: 2 in, 1 out]
                                n336 = local write "D (Rate) Sollwert"(w1178) -> ()
                                n337 = local write "D (Rate) IstWert"(w1178) -> ()
                                }
                                frame 3 {
                                n338 = String Subset(string=w1183, offset (0)=3) -> (substring=w1184:string)  [unwired: 1 in]
                                n339 = Hexadecimal String To Number(string=w1184) -> (number=w1182:u32)  [unwired: 2 in, 1 out]
                                n340 = local write "% LOW Istwert"(w1182) -> ()
                                n341 = local write "% LOW Sollwert"(w1182) -> ()
                                }
                                frame 4 {
                                n342 = String Subset(string=w1187, offset (0)=3) -> (substring=w1188:string)  [unwired: 1 in]
                                n343 = Hexadecimal String To Number(string=w1188) -> (number=w1186:u32)  [unwired: 2 in, 1 out]
                                n344 = local write "% High Sollwert"(w1186) -> ()
                                n345 = local write "% HIGH Istwert"(w1186) -> ()
                                }
                                frame 5 {
                                n346 = call "I3252_Edit_Setpoint.vi"("Read String"=w1191) -> ("Setpoint is"=w1190:dbl)
                                n347 = local write "SP 1 is (°C)"(w1190) -> ()
                                }
                              }
                            }
                          }
                        }
                      }
                      frame #2 {
                        n348 = property on="Get Values" class="Bool"("Blinking"=FALSE) -> ()  [unwired: 2 in, 2 out]
                      }
                    }
                    n349 = Not(x="Get Values") -> (.not. x?=w1126:bool)
                    n350 = Unbundle(w1121) -> ("VISA resource name out"=w1120:refnum<visa-resource-name>, "error out"=w1119:errorcluster)  [unwired: 2 out]
                  }
                  event "Get Values 2": Value Change {
                    n351 = event-data() -> ()  [unwired: 1 in, 1 out]
                    n352 = stacked-sequence {
                      tunnel: w1195 -> [_ w1205 _]
                      tunnel: [_ w1204 _] -> w1194
                      tunnel: [_ w1203 _] -> w1193
                      frame #0 {
                        n353 = property on="Get Values 2" class="Bool"("Blinking"=TRUE) -> ()  [unwired: 2 in, 2 out]
                        n354 = property on="ON 2" class="Bool (strict)"("Blinking"=FALSE) -> ()  [unwired: 2 in, 2 out]
                      }
                      frame #1 {
                        n355 = for {
                          N: 6 -> [_]
                          tunnel: w1205 -> [w1209]
                          tunnel: [w1208] -> w1204
                          tunnel: [w1207] -> w1203
                          i -> [w1211]
                          n356 = flat-sequence {
                            tunnel: w1211 -> [w1213]
                            tunnel: [w1214] -> w1210
                            tunnel: w1210 -> [w1236]
                            tunnel: [w1237] -> w1212
                            tunnel: w1209 -> [w1235]
                            tunnel: [w1234] -> w1207
                            tunnel: [w1233] -> w1208
                            tunnel: w1212 -> [w1243]
                            tunnel: w1211 -> [w1242]
                            frame #0 {
                              n357 = case shown="1" w1213 {
                                tunnel: [w1217 w1221 w1225 "*R27" "*R28" w1231] -> w1214
                                frame 0, Default {
                                n358 = local read "RAM 2"() -> (w1218:bool)
                                n359 = Select(t="*G17", s=w1218, f="*R17") -> (s? t:f=w1217:string)
                                }
                                frame 1 {
                                n360 = local read "RAM 2"() -> (w1222:bool)
                                n361 = Select(t="*G18", s=w1222, f="*R18") -> (s? t:f=w1221:string)
                                }
                                frame 2 {
                                n362 = local read "RAM 2"() -> (w1226:bool)
                                n363 = Select(t="*G19", s=w1226, f="*R19") -> (s? t:f=w1225:string)
                                }
                                frame 3 {
                                }
                                frame 4 {
                                }
                                frame 5 {
                                n364 = local read "RAM 2"() -> (w1232:bool)
                                n365 = Select(t="*G01", s=w1232, f="*R01") -> (s? t:f=w1231:string)
                                }
                              }
                            }
                            frame #1 {
                              n366 = Unbundle(w1235) -> ("VISA resource name out"=w1241:refnum<visa-resource-name>, "error out"=w1239:errorcluster, "Delay (ms) 2"=w1240:u32, "Write/\nRead \n\n2"=w1238:bool)
                              n367 = call "I3252_Comm_Interface.vi"("VISA resource name in"=w1241, "error in"=w1239, "Delay (ms)"=w1240, "Write"=w1238, "String to Write"=w1236, "Read"=w1238) -> ("VISA resource name out"=w1233:refnum<visa-resource-name>, "error out"=w1234:errorcluster, "Read String"=w1237:string)  [unwired: 2 in]
                            }
                            frame #2 {
                              n368 = case shown="0, Default" w1242 {
                                tunnel: w1243 -> [w1245 w1249 w1253 w1257 w1261 w1265]
                                frame 0, Default {
                                n369 = String Subset(string=w1245, offset (0)=3) -> (substring=w1246:string)  [unwired: 1 in]
                                n370 = Hexadecimal String To Number(string=w1246) -> (number=w1244:u32)  [unwired: 2 in, 1 out]
                                n371 = local write "P (PB1) Sollwert 2"(w1244) -> ()
                                n372 = local write "P (PB1) Istwert 2"(w1244) -> ()
                                }
                                frame 1 {
                                n373 = String Subset(string=w1249, offset (0)=3) -> (substring=w1250:string)  [unwired: 1 in]
                                n374 = Hexadecimal String To Number(string=w1250) -> (number=w1248:u32)  [unwired: 2 in, 1 out]
                                n375 = local write "I ( Reset1) Sollwert 2"(w1248) -> ()
                                n376 = local write "I ( Reset1) Istwert 2"(w1248) -> ()
                                }
                                frame 2 {
                                n377 = String Subset(string=w1253, offset (0)=3) -> (substring=w1254:string)  [unwired: 1 in]
                                n378 = Hexadecimal String To Number(string=w1254) -> (number=w1252:u32)  [unwired: 2 in, 1 out]
                                n379 = local write "D (Rate) Sollwert 2"(w1252) -> ()
                                n380 = local write "D (Rate) IstWert 2"(w1252) -> ()
                                }
                                frame 3 {
                                n381 = String Subset(string=w1257, offset (0)=3) -> (substring=w1258:string)  [unwired: 1 in]
                                n382 = Hexadecimal String To Number(string=w1258) -> (number=w1256:u32)  [unwired: 2 in, 1 out]
                                n383 = local write "% LOW Istwert 2"(w1256) -> ()
                                n384 = local write "% LOW Sollwert 2"(w1256) -> ()
                                }
                                frame 4 {
                                n385 = String Subset(string=w1261, offset (0)=3) -> (substring=w1262:string)  [unwired: 1 in]
                                n386 = Hexadecimal String To Number(string=w1262) -> (number=w1260:u32)  [unwired: 2 in, 1 out]
                                n387 = local write "% High Sollwert 2"(w1260) -> ()
                                n388 = local write "% HIGH Istwert 2"(w1260) -> ()
                                }
                                frame 5 {
                                n389 = call "I3252_Edit_Setpoint.vi"("Read String"=w1265) -> ("Setpoint is"=w1264:dbl)
                                n390 = local write "SP 2 is (°C)"(w1264) -> ()
                                }
                              }
                            }
                          }
                        }
                      }
                      frame #2 {
                        n391 = property on="Get Values 2" class="Bool"("Blinking"=FALSE) -> ()  [unwired: 2 in, 2 out]
                      }
                    }
                    n392 = Not(x="Get Values 2") -> (.not. x?=w1200:bool)
                    n393 = Unbundle(w1196) -> ("VISA resource name out"=w1198:refnum<visa-resource-name>, "error out"=w1197:errorcluster)  [unwired: 2 out]
                  }
                  event "RAM": Value Change {
                    n394 = event-data() -> ()  [unwired: 1 in, 1 out]
                    n395 = stacked-sequence {
                      tunnel: w1272 -> [_ w1279 _]
                      tunnel: [_ w1278 _] -> w1271
                      tunnel: [_ w1277 _] -> w1270
                      frame #0 {
                        n396 = property on="RAM" class="Bool (strict)"("Blinking"=TRUE) -> ()  [unwired: 2 in, 2 out]
                        n397 = property on="ON" class="Bool (strict)"("Blinking"=FALSE) -> ()  [unwired: 2 in, 2 out]
                      }
                      frame #1 {
                        n398 = for {
                          N: 6 -> [_]
                          tunnel: w1279 -> [w1283]
                          tunnel: [w1282] -> w1278
                          tunnel: [w1281] -> w1277
                          i -> [w1285]
                          n399 = flat-sequence {
                            tunnel: w1285 -> [w1287]
                            tunnel: [w1288] -> w1284
                            tunnel: w1284 -> [w1307]
                            tunnel: [w1308] -> w1286
                            tunnel: w1283 -> [w1311]
                            tunnel: [w1310] -> w1281
                            tunnel: [w1309] -> w1282
                            tunnel: w1286 -> [w1317]
                            tunnel: w1285 -> [w1316]
                            frame #0 {
                              n400 = case shown="3" w1287 {
                                tunnel: [w1291 w1295 w1299 "*R27" "*R28" w1305] -> w1288
                                frame 0, Default {
                                n401 = local read "RAM"() -> (w1292:bool)
                                n402 = Select(t="*G17", s=w1292, f="*R17") -> (s? t:f=w1291:string)
                                }
                                frame 1 {
                                n403 = local read "RAM"() -> (w1296:bool)
                                n404 = Select(t="*G18", s=w1296, f="*R18") -> (s? t:f=w1295:string)
                                }
                                frame 2 {
                                n405 = local read "RAM"() -> (w1300:bool)
                                n406 = Select(t="*G19", s=w1300, f="*R19") -> (s? t:f=w1299:string)
                                }
                                frame 3 {
                                }
                                frame 4 {
                                }
                                frame 5 {
                                n407 = local read "RAM"() -> (w1306:bool)
                                n408 = Select(t="*G01", s=w1306, f="*R01") -> (s? t:f=w1305:string)
                                }
                              }
                            }
                            frame #1 {
                              n409 = Unbundle(w1311) -> ("VISA resource name out"=w1315:refnum<visa-resource-name>, "error out"=w1313:errorcluster, "Delay (ms)"=w1314:u32, "Write/\nRead"=w1312:bool)
                              n410 = call "I3252_Comm_Interface.vi"("VISA resource name in"=w1315, "error in"=w1313, "Delay (ms)"=w1314, "Write"=w1312, "String to Write"=w1307, "Read"=w1312) -> ("VISA resource name out"=w1309:refnum<visa-resource-name>, "error out"=w1310:errorcluster, "Read String"=w1308:string)  [unwired: 2 in]
                            }
                            frame #2 {
                              n411 = case shown="5" w1316 {
                                tunnel: w1317 -> [w1319 w1323 w1327 w1331 w1335 w1339]
                                frame 0, Default {
                                n412 = String Subset(string=w1319, offset (0)=3) -> (substring=w1320:string)  [unwired: 1 in]
                                n413 = Hexadecimal String To Number(string=w1320) -> (number=w1318:u32)  [unwired: 2 in, 1 out]
                                n414 = local write "P (PB1) Sollwert"(w1318) -> ()
                                n415 = local write "P (PB1) Istwert"(w1318) -> ()
                                }
                                frame 1 {
                                n416 = String Subset(string=w1323, offset (0)=3) -> (substring=w1324:string)  [unwired: 1 in]
                                n417 = Hexadecimal String To Number(string=w1324) -> (number=w1322:u32)  [unwired: 2 in, 1 out]
                                n418 = local write "I ( Reset1) Sollwert"(w1322) -> ()
                                n419 = local write "I ( Reset1) Istwert"(w1322) -> ()
                                }
                                frame 2 {
                                n420 = String Subset(string=w1327, offset (0)=3) -> (substring=w1328:string)  [unwired: 1 in]
                                n421 = Hexadecimal String To Number(string=w1328) -> (number=w1326:u32)  [unwired: 2 in, 1 out]
                                n422 = local write "D (Rate) IstWert"(w1326) -> ()
                                n423 = local write "D (Rate) Sollwert"(w1326) -> ()
                                }
                                frame 3 {
                                n424 = String Subset(string=w1331, offset (0)=3) -> (substring=w1332:string)  [unwired: 1 in]
                                n425 = Hexadecimal String To Number(string=w1332) -> (number=w1330:u32)  [unwired: 2 in, 1 out]
                                n426 = local write "% LOW Istwert"(w1330) -> ()
                                n427 = local write "% LOW Sollwert"(w1330) -> ()
                                }
                                frame 4 {
                                n428 = String Subset(string=w1335, offset (0)=3) -> (substring=w1336:string)  [unwired: 1 in]
                                n429 = Hexadecimal String To Number(string=w1336) -> (number=w1334:u32)  [unwired: 2 in, 1 out]
                                n430 = local write "% HIGH Istwert"(w1334) -> ()
                                n431 = local write "% High Sollwert"(w1334) -> ()
                                }
                                frame 5 {
                                n432 = call "I3252_Edit_Setpoint.vi"("Read String"=w1339) -> ("Setpoint is"=w1338:dbl)
                                n433 = local write "SP 1 is (°C)"(w1338) -> ()
                                }
                              }
                            }
                          }
                        }
                      }
                      frame #2 {
                        n434 = property on="RAM" class="Bool (strict)"("Blinking"=FALSE) -> ()  [unwired: 2 in, 2 out]
                      }
                    }
                    n435 = Not(x="RAM") -> (.not. x?=w1274:bool)
                    n436 = Unbundle(w1269) -> ("VISA resource name out"=w1268:refnum<visa-resource-name>, "error out"=w1267:errorcluster)  [unwired: 2 out]
                  }
                  event "RAM 2": Value Change {
                    n437 = event-data() -> ()  [unwired: 1 in, 1 out]
                    n438 = stacked-sequence {
                      tunnel: w1343 -> [_ w1353 _]
                      tunnel: [_ w1352 _] -> w1342
                      tunnel: [_ w1351 _] -> w1341
                      frame #0 {
                        n439 = property on="RAM 2" class="Bool (strict)"("Blinking"=TRUE) -> ()  [unwired: 2 in, 2 out]
                        n440 = property on="ON 2" class="Bool (strict)"("Blinking"=FALSE) -> ()  [unwired: 2 in, 2 out]
                      }
                      frame #1 {
                        n441 = for {
                          N: 6 -> [_]
                          tunnel: w1353 -> [w1357]
                          tunnel: [w1356] -> w1352
                          tunnel: [w1355] -> w1351
                          i -> [w1359]
                          n442 = flat-sequence {
                            tunnel: w1359 -> [w1361]
                            tunnel: [w1362] -> w1358
                            tunnel: w1358 -> [w1381]
                            tunnel: [w1382] -> w1360
                            tunnel: w1357 -> [w1385]
                            tunnel: [w1384] -> w1355
                            tunnel: [w1383] -> w1356
                            tunnel: w1360 -> [w1391]
                            tunnel: w1359 -> [w1390]
                            frame #0 {
                              n443 = case shown="5" w1361 {
                                tunnel: [w1365 w1369 w1373 "*R27" "*R28" w1379] -> w1362
                                frame 0, Default {
                                n444 = local read "RAM 2"() -> (w1366:bool)
                                n445 = Select(t="*G17", s=w1366, f="*R17") -> (s? t:f=w1365:string)
                                }
                                frame 1 {
                                n446 = local read "RAM 2"() -> (w1370:bool)
                                n447 = Select(t="*G18", s=w1370, f="*R18") -> (s? t:f=w1369:string)
                                }
                                frame 2 {
                                n448 = local read "RAM 2"() -> (w1374:bool)
                                n449 = Select(t="*G19", s=w1374, f="*R19") -> (s? t:f=w1373:string)
                                }
                                frame 3 {
                                }
                                frame 4 {
                                }
                                frame 5 {
                                n450 = local read "RAM 2"() -> (w1380:bool)
                                n451 = Select(t="*G01", s=w1380, f="*R01") -> (s? t:f=w1379:string)
                                }
                              }
                            }
                            frame #1 {
                              n452 = Unbundle(w1385) -> ("VISA resource name out"=w1389:refnum<visa-resource-name>, "error out"=w1387:errorcluster, "Delay (ms) 2"=w1388:u32, "Write/\nRead \n\n2"=w1386:bool)
                              n453 = call "I3252_Comm_Interface.vi"("VISA resource name in"=w1389, "error in"=w1387, "Delay (ms)"=w1388, "Write"=w1386, "String to Write"=w1381, "Read"=w1386) -> ("VISA resource name out"=w1383:refnum<visa-resource-name>, "error out"=w1384:errorcluster, "Read String"=w1382:string)  [unwired: 2 in]
                            }
                            frame #2 {
                              n454 = case shown="0, Default" w1390 {
                                tunnel: w1391 -> [w1393 w1397 w1401 w1405 w1409 w1413]
                                frame 0, Default {
                                n455 = String Subset(string=w1393, offset (0)=3) -> (substring=w1394:string)  [unwired: 1 in]
                                n456 = Hexadecimal String To Number(string=w1394) -> (number=w1392:u32)  [unwired: 2 in, 1 out]
                                n457 = local write "P (PB1) Sollwert 2"(w1392) -> ()
                                n458 = local write "P (PB1) Istwert 2"(w1392) -> ()
                                }
                                frame 1 {
                                n459 = String Subset(string=w1397, offset (0)=3) -> (substring=w1398:string)  [unwired: 1 in]
                                n460 = Hexadecimal String To Number(string=w1398) -> (number=w1396:u32)  [unwired: 2 in, 1 out]
                                n461 = local write "I ( Reset1) Sollwert 2"(w1396) -> ()
                                n462 = local write "I ( Reset1) Istwert 2"(w1396) -> ()
                                }
                                frame 2 {
                                n463 = String Subset(string=w1401, offset (0)=3) -> (substring=w1402:string)  [unwired: 1 in]
                                n464 = Hexadecimal String To Number(string=w1402) -> (number=w1400:u32)  [unwired: 2 in, 1 out]
                                n465 = local write "D (Rate) IstWert 2"(w1400) -> ()
                                n466 = local write "D (Rate) Sollwert 2"(w1400) -> ()
                                }
                                frame 3 {
                                n467 = String Subset(string=w1405, offset (0)=3) -> (substring=w1406:string)  [unwired: 1 in]
                                n468 = Hexadecimal String To Number(string=w1406) -> (number=w1404:u32)  [unwired: 2 in, 1 out]
                                n469 = local write "% LOW Istwert 2"(w1404) -> ()
                                n470 = local write "% LOW Sollwert 2"(w1404) -> ()
                                }
                                frame 4 {
                                n471 = String Subset(string=w1409, offset (0)=3) -> (substring=w1410:string)  [unwired: 1 in]
                                n472 = Hexadecimal String To Number(string=w1410) -> (number=w1408:u32)  [unwired: 2 in, 1 out]
                                n473 = local write "% HIGH Istwert 2"(w1408) -> ()
                                n474 = local write "% High Sollwert 2"(w1408) -> ()
                                }
                                frame 5 {
                                n475 = call "I3252_Edit_Setpoint.vi"("Read String"=w1413) -> ("Setpoint is"=w1412:dbl)
                                n476 = local write "SP 2 is (°C)"(w1412) -> ()
                                }
                              }
                            }
                          }
                        }
                      }
                      frame #2 {
                        n477 = property on="RAM 2" class="Bool (strict)"("Blinking"=FALSE) -> ()  [unwired: 2 in, 2 out]
                      }
                    }
                    n478 = Not(x="RAM 2") -> (.not. x?=w1348:bool)
                    n479 = Unbundle(w1346) -> ("VISA resource name out"=w1345:refnum<visa-resource-name>, "error out"=w1344:errorcluster)  [unwired: 2 out]
                  }
                  event "Set Gauge to Zero": Value Change {
                    n480 = event-data() -> ()  [unwired: 1 in, 1 out]
                    n481 = flat-sequence {
                      tunnel: w1422 -> [w1427]
                      tunnel: [w1427] -> w1421
                      tunnel: w1421 -> [w1429]
                      tunnel: [w1433] -> w1420
                      tunnel: [w1432] -> w1419
                      tunnel: [w1429] -> w1418
                      tunnel: w1420 -> [w1439]
                      tunnel: w1419 -> [w1438]
                      tunnel: w1418 -> [w1434]
                      frame #0 {
                        n482 = property on="Set Gauge to Zero" class="Bool"("Blinking"=TRUE) -> ()  [unwired: 2 in, 2 out]
                      }
                      frame #1 {
                        w1430 = 0 items=["sensor 1", "sensor 2", "test"] ("Sensor Nr.:")
                        n483 = call "DUAL GAUGE-Get Pressure,Status.vi"("Sensor Nr.:"=w1430, "Referenz in"=w1429) -> ("Pressure"=w1433:dbl)  [unwired: 6 in, 3 out]
                        n484 = call "DUAL GAUGE-Offset display.vi"("W/R"=FALSE, "Referenz in"=w1429) -> ("Sensor 1 Get"=w1432:dbl)  [unwired: 6 in, 3 out]
                      }
                      frame #2 {
                        n485 = Add(x=w1439, y=w1438) -> (x+y=w1435:dbl)
                        n486 = call "DUAL GAUGE-Offset display.vi"("W/R"=TRUE, "Sensor 1 Set"=w1435, "Referenz in"=w1434) -> ("Sensor 1 Get"=→"Current Offset (mbar)":dbl)  [unwired: 5 in, 3 out]
                      }
                      frame #3 {
                        n487 = property on="Set Gauge to Zero" class="Bool"("Blinking"=TRUE) -> ()  [unwired: 2 in, 2 out]
                      }
                    }
                    n488 = Unbundle(w1426) -> ("VISA resource name out"=w1425:refnum<visa-resource-name>, "error out"=w1424:errorcluster)  [unwired: 2 out]
                    n489 = Unbundle(w1417) -> ("VISA resource name out"=w1416:refnum<visa-resource-name>, "error out"=w1415:errorcluster)  [unwired: 2 out]
                  }
                  event "Write to File": Value Change {
                    n490 = event-data() -> ("NewVal"=w1448:bool)  [unwired: 1 in]
                    n491 = Unbundle(w1451) -> ("VISA resource name out"=w1450:refnum<visa-resource-name>, "error out"=w1449:errorcluster)  [unwired: 2 out]
                    n492 = local read "File Path"() -> (w1444:path)
                    n493 = case shown="False" w1448 {
                      tunnel: w1444 -> [_ w1456]
                      tunnel: "User" -> [_ w1455]
                      tunnel: "Sample" -> [_ w1454]
                      tunnel: [path "" ("File Path") w1453] -> w1445
                      frame False {
                      }
                      frame True {
                        n494 = call "Header.vi"("Sample"=w1454, "User"=w1455, "File Path"=w1456) -> ("File Path"=w1453:path)
                      }
                    }
                    n495 = local write "File Path"(w1445) -> ()
                    n496 = Unbundle(w1443) -> ("VISA resource name out"=w1442:refnum<visa-resource-name>, "error out"=w1441:errorcluster)  [unwired: 2 out]
                  }
                }
              }
              n497 = Bundle(cluster=w426, "VISA resource name out"=w425, "error out"=w424) -> (w423:T7)  [unwired: 2 in]
              n498 = Bundle(cluster=w402, "VISA resource name out"=w404, "error out"=w403) -> (w401:T8)  [unwired: 2 in]
            }
            frame #2 {
            }
            frame #3 {
              (unwired) "Daniel Schuster (geb. 20.03.1988)"
              n499 = node-c288(w1518) -> (w1527:T3)  [unwired: 2 in]
              n500 = node-c288(w1533) -> (w1536:T3)  [unwired: 2 in]
              n501 = node-c288(w1523) -> (w1525:T3)  [unwired: 2 in]
              n502 = node-c288(w1532) -> (w1540:T3)  [unwired: 2 in]
              n503 = timed-sequence {
                timing: w1527 -> [_]
                timing-out: [_] -> w1526
                tunnel: w1502 -> [w1612]
                tunnel: w1501 -> [w1608]
                tunnel: [w1611] -> w1494
                tunnel: w1493 -> [w1610]
                tunnel: w1492 -> [w1609]
                tunnel: [w1607] -> w1491
                tunnel: [w1606] -> w1490
                tunnel: [w1605] -> w1488
                n504 = timed-flat-sequence {
                  tunnel: w1612 -> [w1621]
                  tunnel: [w1620] -> w1611
                  tunnel: w1610 -> [w1619]
                  tunnel: w1609 -> [w1618]
                  tunnel: w1608 -> [w1617]
                  tunnel: [w1615] -> w1607
                  tunnel: [w1614] -> w1606
                  tunnel: [w1613] -> w1605
                  n505 = node-c288() -> ()  [unwired: 1 in, 1 out]
                  n506 = case shown="True" "ON (TPG 2)" {
                    tunnel: w1617 -> [w1626 w1632]
                    tunnel: w1618 -> [w1625 w1631]
                    tunnel: [w1624 w1630] -> w1614
                    tunnel: [w1623 w1629] -> w1613
                    frame False {
                      w1627 = 0.0 ("Pressure")
                      n507 = property on="ON (TPG 2)" class="Bool (strict)"("Blinking"=FALSE) -> ()  [unwired: 2 in, 2 out]
                      n508 = Bundle("Pressure"=w1627, "Pressure"=w1627) -> (w1624:cluster{"Pressure":dbl, "Pressure":dbl})  [unwired: 1 in]
                      n509 = Bundle("TPG 2 COM"=w1626, "error out"=w1625) -> (w1623:T9)  [unwired: 1 in]
                    }
                    frame True {
                      n510 = stacked-sequence {
                        tunnel: w1632 -> [_ w1645]
                        tunnel: [_ w1641] -> w1630
                        tunnel: [_ w1637] -> w1629
                        tunnel: w1631 -> [_ w1634]
                        frame #0 {
                          n511 = property on="ON (TPG 2)" class="Bool (strict)"("Blinking"=TRUE) -> ()  [unwired: 2 in, 2 out]
                        }
                        frame #1 {
                          n512 = call "PresureGetSubVI.vi"("COM in"=w1645, "Fehler (Eingang)"=w1634) -> ("Status Gauge#1"=→"Status Gauge 2#1":i32, "Status Gauge#2"=→"Status Gauge 2#2":i32, "COM out"=w1638:refnum<visa-resource-name>, "Pressure Gauge#1"=w1639:dbl, "Pressure Gauge#2"=w1642:dbl, "Cluster (Ausgang)"=w1635:errorcluster)  [unwired: 12 in]
                          "Pressure Gauge 2#1" <- w1639
                          "Pressure Gauge 2#2" <- w1642
                          n513 = Bundle("COM out"=w1638, "Cluster (Ausgang)"=w1635) -> (w1637:T10)  [unwired: 1 in]
                          n514 = Unbundle(w1635) -> ("status"=w1636:bool, "code"=w1640:i32)  [unwired: 1 out]
                          n515 = Bundle("status"=w1636, "code"=w1640) -> ()  [unwired: 1 in, 1 out]
                          n516 = Bundle("Pressure Gauge#1"=w1639, "Pressure Gauge#2"=w1642) -> (w1641:T11)  [unwired: 1 in]
                        }
                      }
                    }
                  }
                  n517 = case shown="True" "ON (TPG 1)" {
                    tunnel: w1621 -> [w1649 w1655]
                    tunnel: [w1648 w1654] -> w1620
                    tunnel: w1619 -> [w1647 w1653]
                    tunnel: [w1646 w1652] -> w1615
                    frame False {
                      w1650 = 0.0 ("Pressure")
                      n518 = property on="ON (TPG 1)" class="Bool (strict)"("Blinking"=FALSE) -> ()  [unwired: 2 in, 2 out]
                      n519 = Bundle("Pressure"=w1650, "Pressure"=w1650) -> (w1646:cluster{"Pressure":dbl, "Pressure":dbl})  [unwired: 1 in]
                      n520 = Bundle("TPG 1 COM"=w1649, "error out"=w1647) -> (w1648:T12)  [unwired: 1 in]
                    }
                    frame True {
                      n521 = stacked-sequence {
                        tunnel: w1655 -> [_ w1668]
                        tunnel: [_ w1661] -> w1654
                        tunnel: w1653 -> [_ w1658]
                        tunnel: [_ w1657] -> w1652
                        frame #0 {
                          n522 = property on="ON (TPG 1)" class="Bool (strict)"("Blinking"=TRUE) -> ()  [unwired: 2 in, 2 out]
                        }
                        frame #1 {
                          n523 = call "PresureGetSubVI.vi"("COM in"=w1668, "Fehler (Eingang)"=w1658) -> ("Status Gauge#1"=→"Status Gauge 1#1":i32, "Status Gauge#2"=→"Status Gauge 1#2":i32, "COM out"=w1662:refnum<visa-resource-name>, "Pressure Gauge#1"=w1663:dbl, "Pressure Gauge#2"=w1665:dbl, "Cluster (Ausgang)"=w1659:errorcluster)  [unwired: 12 in]
                          "Pressure Gauge 1#1" <- w1663
                          "Pressure Gauge 1#2" <- w1665
                          n524 = Bundle("COM out"=w1662, "Cluster (Ausgang)"=w1659) -> (w1661:T10)  [unwired: 1 in]
                          n525 = Unbundle(w1659) -> ("status"=w1660:bool, "code"=w1664:i32)  [unwired: 1 out]
                          n526 = Bundle("status"=w1660, "code"=w1664) -> ()  [unwired: 1 in, 1 out]
                          n527 = Bundle("Pressure Gauge#1"=w1663, "Pressure Gauge#2"=w1665) -> (w1657:T11)  [unwired: 1 in]
                        }
                      }
                    }
                  }
                  n528 = node-c288() -> ()  [unwired: 1 in, 1 out]
                }
              }
              n529 = timed-sequence {
                timing: w1536 -> [_]
                timing-out: [_] -> w1535
                tunnel: w1534 -> [w1678]
                tunnel: [w1677] -> w1529
                tunnel: [w1676] -> w1528
                tunnel: [w1675] -> w1515
                n530 = timed-flat-sequence {
                  tunnel: w1678 -> [w1682]
                  tunnel: [w1681] -> w1677
                  tunnel: [w1680] -> w1676
                  tunnel: [w1679] -> w1675
                  n531 = node-c288() -> ()  [unwired: 1 in, 1 out]
                  n532 = case shown="False" "ON" {
                    tunnel: w1682 -> [w1686 w1691]
                    tunnel: [w1685 w1690] -> w1681
                    tunnel: [w1684 w1689] -> w1680
                    tunnel: [_ w1688] -> w1679
                    frame False {
                      n533 = Unbundle(w1686) -> ("VISA resource name out"=w1685:refnum<visa-resource-name>, "error out"=w1684:errorcluster)  [unwired: 2 out]
                      n534 = property on="ON" class="Bool (strict)"("Blinking"=FALSE) -> ()  [unwired: 2 in, 2 out]
                    }
                    frame True {
                      n535 = stacked-sequence {
                        tunnel: w1691 -> [_ w1696]
                        tunnel: [_ w1695] -> w1690
                        tunnel: [_ w1694] -> w1689
                        tunnel: [_ w1693] -> w1688
                        frame #0 {
                          n536 = property on="ON" class="Bool (strict)"("Blinking"=TRUE) -> ()  [unwired: 2 in, 2 out]
                        }
                        frame #1 {
                          n537 = Unbundle(w1696) -> ("VISA resource name out"=w1700:refnum<visa-resource-name>, "error out"=w1698:errorcluster, "Delay (ms)"=w1699:u32, "Write/\nRead"=w1697:bool)
                          n538 = call "I3252_Comm_Interface.vi"("VISA resource name in"=w1700, "error in"=w1698, "Delay (ms)"=w1699, "Write"=w1697, "String to Write"="*V01", "Read"=w1697) -> ("VISA resource name out"=w1695:refnum<visa-resource-name>, "error out"=w1694:errorcluster, "Read String"=w1693:string)  [unwired: 2 in]
                        }
                      }
                    }
                  }
                  n539 = node-c288() -> ()  [unwired: 1 in, 1 out]
                }
              }
              n540 = timed-sequence {
                timing: w1525 -> [_]
                timing-out: [_] -> w1524
                tunnel: w1522 -> [w1574]
                tunnel: w1521 -> [w1573]
                tunnel: [w1572] -> w1519
                tunnel: [w1571] -> w1520
                tunnel: [w1570] -> w1516
                n541 = timed-flat-sequence {
                  tunnel: w1574 -> [w1579]
                  tunnel: w1573 -> [w1578]
                  tunnel: [w1577] -> w1572
                  tunnel: [w1576] -> w1571
                  tunnel: [w1575] -> w1570
                  n542 = node-c288() -> ()  [unwired: 1 in, 1 out]
                  n543 = case shown="False" "ON" {
                    tunnel: w1579 -> [w1583 w1589]
                    tunnel: w1578 -> [w1584 w1588]
                    tunnel: [w1583 w1587] -> w1577
                    tunnel: [w1584 w1586] -> w1576
                    tunnel: [0.0 ("Reading") w1585] -> w1575
                    frame False {
                      n544 = property on="ON" class="Bool (strict)"("Blinking"=FALSE) -> ()  [unwired: 2 in, 2 out]
                    }
                    frame True {
                      n545 = stacked-sequence {
                        tunnel: w1589 -> [_ w1596]
                        tunnel: w1588 -> [_ w1595]
                        tunnel: [_ w1594] -> w1587
                        tunnel: [_ w1593] -> w1586
                        tunnel: [_ w1591] -> w1585
                        frame #0 {
                          n546 = property on="ON" class="Bool (strict)"("Blinking"=TRUE) -> ()  [unwired: 2 in, 2 out]
                        }
                        frame #1 {
                          n547 = call "VC840_Read.vi"("error in (no error)"=w1595, "VISA resource name"=w1596) -> ("error out"=w1593:errorcluster, "Unit"=→"Unit 2":string, "Reading"=w1591:dbl, "VISA resource name out"=w1594:refnum<visa-resource-name>, "Status"=→"Status 2":T2, "Mode"=→"Mode 2":enum16{"?", "Diode", "Beep", "DC", "AC"})  [unwired: 4 out]
                          "Reading 2" <- w1591
                        }
                      }
                    }
                  }
                  n548 = node-c288() -> ()  [unwired: 1 in, 1 out]
                }
              }
              n549 = timed-sequence {
                timing: w1540 -> [_]
                timing-out: [_] -> w1539
                tunnel: w1538 -> [w1712]
                tunnel: w1537 -> [w1711]
                tunnel: [w1710] -> w1531
                tunnel: [w1709] -> w1530
                tunnel: [w1708] -> w1517
                n550 = timed-flat-sequence {
                  tunnel: w1712 -> [w1717]
                  tunnel: w1711 -> [w1716]
                  tunnel: [w1715] -> w1710
                  tunnel: [w1714] -> w1709
                  tunnel: [w1713] -> w1708
                  n551 = node-c288() -> ()  [unwired: 1 in, 1 out]
                  n552 = case shown="True" "ON" {
                    tunnel: w1717 -> [w1721 w1727]
                    tunnel: w1716 -> [w1722 w1726]
                    tunnel: [w1721 w1725] -> w1715
                    tunnel: [w1722 w1724] -> w1714
                    tunnel: [0.0 ("Reading") w1723] -> w1713
                    frame False {
                      n553 = property on="ON" class="Bool (strict)"("Blinking"=FALSE) -> ()  [unwired: 2 in, 2 out]
                    }
                    frame True {
                      n554 = stacked-sequence {
                        tunnel: w1727 -> [_ w1734]
                        tunnel: w1726 -> [_ w1733]
                        tunnel: [_ w1732] -> w1725
                        tunnel: [_ w1731] -> w1724
                        tunnel: [_ w1729] -> w1723
                        frame #0 {
                          n555 = property on="ON" class="Bool (strict)"("Blinking"=TRUE) -> ()  [unwired: 2 in, 2 out]
                        }
                        frame #1 {
                          n556 = call "VC840_Read.vi"("error in (no error)"=w1733, "VISA resource name"=w1734) -> ("error out"=w1731:errorcluster, "Unit"=→"Unit 1":string, "Reading"=w1729:dbl, "VISA resource name out"=w1732:refnum<visa-resource-name>, "Status"=→"Status 1":T2, "Mode"=→"Mode 1":enum16{"?", "Diode", "Beep", "DC", "AC"})  [unwired: 4 out]
                          "Reading 1" <- w1729
                        }
                      }
                    }
                  }
                  n557 = node-c288() -> ()  [unwired: 1 in, 1 out]
                }
              }
              n558 = Tick Count (ms)() -> (millisecond timer value=w1503:u32)
              n559 = Subtract(x=w1503, y=w1508) -> (x-y=w1507:u32)
              n560 = Divide(x=w1507, y=u32 1000) -> (x/y=w1505:dbl)
              n561 = node-c288(w1535) -> ()  [unwired: 1 out]
              n562 = node-c288(w1539) -> ()  [unwired: 1 out]
              n563 = node-c288(w1524) -> ()  [unwired: 1 out]
              n564 = node-c288() -> (w1486:T3)  [unwired: 3 in]
              n565 = To Double Precision Float(number=w1505) -> (double precision float=w1509:dbl)
              "current time (s)" <- w1509
              n566 = timed-sequence {
                timing: w1486 -> [_]
                timing-out: [_] -> w1485
                tunnel: w1484 -> [w1544]
                tunnel: [w1543] -> w1481
                tunnel: [w1542] -> w1480
                tunnel: [w1541] -> w1483
                n567 = timed-flat-sequence {
                  tunnel: w1544 -> [w1549]
                  tunnel: [w1548] -> w1543
                  tunnel: [w1547] -> w1542
                  tunnel: [w1546] -> w1541
                  n568 = node-c288() -> ()  [unwired: 1 in, 1 out]
                  n569 = case shown="True" "ON 2" {
                    tunnel: w1549 -> [w1552 w1556]
                    tunnel: [w1551 w1555] -> w1548
                    tunnel: [w1550 w1554] -> w1547
                    tunnel: [_ w1553] -> w1546
                    frame False {
                      (unwired) FALSE
                      n570 = Unbundle(w1552) -> ("VISA resource name out"=w1551:refnum<visa-resource-name>, "error out"=w1550:errorcluster)  [unwired: 2 out]
                    }
                    frame True {
                      n571 = stacked-sequence {
                        tunnel: w1556 -> [_ w1560]
                        tunnel: [_ w1559] -> w1555
                        tunnel: [_ w1558] -> w1554
                        tunnel: [_ w1557] -> w1553
                        frame #0 {
                          (unwired) TRUE
                        }
                        frame #1 {
                          n572 = Unbundle(w1560) -> ("VISA resource name out"=w1564:refnum<visa-resource-name>, "error out"=w1562:errorcluster, "Delay (ms) 2"=w1563:u32, "Write/\nRead \n\n2"=w1561:bool)
                          n573 = call "I3252_Comm_Interface.vi"("VISA resource name in"=w1564, "error in"=w1562, "Delay (ms)"=w1563, "Write"=w1561, "String to Write"="*V01", "Read"=w1561) -> ("VISA resource name out"=w1559:refnum<visa-resource-name>, "error out"=w1558:errorcluster, "Read String"=w1557:string)  [unwired: 2 in]
                        }
                      }
                    }
                  }
                  n574 = node-c288() -> ()  [unwired: 1 in, 1 out]
                }
              }
              n575 = node-c288(w1526) -> ()  [unwired: 1 out]
              n576 = Unbundle(w1490) -> ("Pressure Gauge#1"=w1489:dbl, "Pressure Gauge#2"=w1487:dbl)
              "Pressure OpenPort2" <- w1487
              "Pressure Pirani 2" <- w1489
              n577 = Unbundle(w1491) -> ("Pressure Gauge#1"=w1500:dbl, "Pressure Gauge#2"=w1495:dbl)
              "Pressure Baratron 2" <- w1500
              "Pressure FullRange 2" <- w1495
              n578 = node-c288(w1485) -> ()  [unwired: 1 out]
            }
            frame #4 {
              n579 = Build Array (concatenate)(w1760, w1764) -> (w1759:dbl[])
              n580 = Build Array (concatenate)(w1763, w1765) -> (w1758:dbl[])
              n581 = Build Array (concatenate)(w1761, w1752) -> (w1756:dbl[])
              n582 = Build Array (concatenate)(w1762, w1753) -> (w1757:dbl[])
              n583 = Greater?(x=w1784, y="Pressure Limit (mbar)") -> (0:w1787:bool)
              n584 = case shown="False" w1787 {
                frame False {
                  n585 = property on="Standby" class="Bool (strict)"("DisabledEnum"=T6."Enabled" ("Disabled")) -> ()  [unwired: 2 in, 2 out]
                }
                frame True {
                  n586 = property on="Standby" class="Bool (strict)"("Val(Sgnl)"=TRUE ("Standby"), "DisabledEnum"=T6."Disabled" ("Disabled")) -> ()  [unwired: 2 in, 2 out]
                }
              }
              n587 = call "Resistivity_Calculation.vi"("Reading 1 (V)"=w1777, "Constant"="4PP constant", "Thickness (nm)"="Thickness (nm)", "Reading 2 (A)"=w1785) -> ("Resivtivity (Ohm*cm)"=w1769:dbl, "Current"=w1770:dbl, "Voltage"=w1771:dbl)
              "Resistivity (Ohm*cm)" <- w1769
              "Voltage (V)" <- w1771
              "Current (A)" <- w1770
              n588 = call "I3252_Edit_Temperature.vi"("Temp. String"=w1786) -> ("Temp. (°C)"=w1780:dbl)
              "(°C)" <- w1780
              n589 = call "I3252_Edit_Temperature.vi"("Temp. String"=w1748) -> ("Temp. (°C)"=w1747:dbl)
              "(°C) 2" <- w1747
              n590 = Build Array (concatenate)(w1782, w1783) -> (w1779:dbl[])
              n591 = Build Array (concatenate)(w1781, w1780) -> (w1767:dbl[])
              n592 = Build Array (concatenate)(w1745, w1747) -> (w1746:dbl[])
              n593 = Build Array (concatenate)(w1778, w1771) -> (w1776:dbl[])
              n594 = Build Array (concatenate)(w1775, w1770) -> (w1773:dbl[])
              n595 = Build Array (concatenate)(w1774, w1769) -> (w1772:dbl[])
              n596 = Build Array(w1771, w1770, w1769) -> (w1768:dbl[])
            }
            frame #5 {
              n597 = Bundle(w1802, w1819) -> (→"CMR275 Baratron":cluster{dbl[], dbl[]})  [unwired: 1 in]
              n598 = Bundle(w1802, w1818) -> (→"PKR251 FullRange":cluster{dbl[], dbl[]})  [unwired: 1 in]
              n599 = Bundle(w1802, w1817) -> (→"Pirani (VVP1 Scroll)":cluster{dbl[], dbl[]})  [unwired: 1 in]
              n600 = Bundle(w1802, w1816) -> (→"Pressure OpenPort":cluster{dbl[], dbl[]})  [unwired: 1 in]
              n601 = Bundle(w1802, w1825) -> (→"Thermocouple (Sample holder 1)":cluster{dbl[], dbl[]})  [unwired: 1 in]
              n602 = Bundle(w1802, w1827) -> (→"Voltage":cluster{dbl[], dbl[]})  [unwired: 1 in]
              n603 = Bundle(w1802, w1828) -> (→"Current":cluster{dbl[], dbl[]})  [unwired: 1 in]
              n604 = Bundle(w1802, w1829) -> (→"Resistivity":cluster{dbl[], dbl[]})  [unwired: 1 in]
              n605 = Bundle(w1802, w1803) -> (→"Thermocouple (Sample holder 1) 2":cluster{dbl[], dbl[]})  [unwired: 1 in]
              n606 = Build Array (concatenate)(w1824, w1834, w1833, w1823, w1811, w1807, w1805) -> (w1841:dbl[])
              "appended array" <- w1841
            }
            frame #6 {
              n607 = Unbundle(w1850) -> ("COM out"=w1849:refnum<visa-resource-name>, "Cluster (Ausgang)"=w1848:errorcluster)
              n608 = Unbundle(w1847) -> ("COM out"=w1846:refnum<visa-resource-name>, "Cluster (Ausgang)"=w1845:errorcluster)
              n609 = case shown="True" "Write to File" {
                tunnel: [_ w1878] -> w1864
                tunnel: "File Path" -> [_ w1876]
                tunnel: w1857 -> [_ w1874]
                frame False {
                  n610 = property on="Write to File" class="Bool (strict)"("Blinking"=FALSE) -> ()  [unwired: 2 in, 2 out]
                }
                frame True {
                  n611 = flat-sequence {
                    tunnel: [w1880] -> w1877
                    tunnel: w1876 -> [w1880]
                    tunnel: [w1879] -> w1875
                    tunnel: w1874 -> [w1879]
                    tunnel: [w1885] -> w1878
                    tunnel: w1877 -> [w1884]
                    tunnel: w1875 -> [w1883]
                    frame #0 {
                      n612 = property on="Write to File" class="Bool (strict)"("Blinking"=TRUE) -> ()  [unwired: 2 in, 2 out]
                    }
                    frame #1 {
                      n613 = call-poly <vilib>:"Write To Spreadsheet File.vi"("format (%.3f)"="%g", "append to file? (new file:F)"=TRUE ("transpose? (no:F)"), "1D data"=w1883, "file path (dialog if empty)"=w1884) -> ("new file path (Not A Path if cancelled)"=w1885:path)  [unwired: 4 in]
                    }
                  }
                }
              }
              n614 = Merge Errors(w1869, w1868, w1866, w1848, w1845) -> (w1867:errorcluster)
              n615 = call <vilib>:"Simple Error Handler.vi"("error in (no error)"=w1867) -> ("error?"=w1851:bool)  [unwired: 4 in, 4 out]
              n616 = local write "File Path"(w1864) -> ()
            }
            frame #7 {
              w1904 = u32 1000 ("y")
              n617 = Tick Count (ms)() -> (millisecond timer value=w1906:u32)
              n618 = Subtract(x=w1906, y=w1905) -> (x-y=w1907:u32)
              n619 = VISA Flush I/O Buffer(VISA resource name=w1898, error in (no error)=w1897) -> (VISA resource name out=w1895:refnum<visa-resource-name>, error out=w1896:errorcluster)  [unwired: 1 in]
              n620 = VISA Flush I/O Buffer(VISA resource name=w1891, error in (no error)=w1890) -> (VISA resource name out=w1894:refnum<visa-resource-name>, error out=w1893:errorcluster)  [unwired: 1 in]
              n621 = Divide(x=w1907, y=w1904) -> (x/y=→"loop time (s)":dbl)
              n622 = Subtract(x="Intervall (s)", y=u32 1) -> (x-y=w1908:u32)
              n623 = Multiply(x=w1908, y=w1904) -> (x*y=w1911:u32)
              n624 = Wait (ms)(milliseconds to wait=w1911) -> ()  [unwired: 1 out]
              n625 = Bundle("COM out"=w1895, "error out"=w1896, "COM out"=w1894, "error out"=w1893) -> (w1892:T13)  [unwired: 1 in]
            }
            frame #8 {
              n626 = Tick Count (ms)() -> (millisecond timer value=w1934:u32)
              n627 = Subtract(x=w1934, y=w1932) -> (x-y=w1933:u32)
              n628 = Divide(x=w1933, y=w1931) -> (x/y=→"data logger intervall (s)":dbl)
            }
          }
          n629 = Exclusive Or(1:"stop", 2:w183) -> (0:w184:bool)
        }
      }
      frame #4 {
        n630 = call "VC840_Close.vi"("error in (no error)"=w1956, "VISA resource name"=w1957) -> ("error out"=w1965:errorcluster)  [unwired: 9 in]
        n631 = call "VC840_Close.vi"("error in (no error)"=w1958, "VISA resource name"=w1959) -> ("error out"=w1963:errorcluster)  [unwired: 9 in]
        n632 = VISA Close(VISA resource name=w1961, error in (no error)=w1960) -> (error out=w1962:errorcluster)
        n633 = VISA Close(VISA resource name=w1949, error in (no error)=w1948) -> (error out=w1947:errorcluster)
        n634 = Unbundle(w1954) -> ("COM out"=w1953:refnum<visa-resource-name>, "error out"=w1952:errorcluster, "COM out"=w1950:refnum<visa-resource-name>, "error out"=w1951:errorcluster)
        n635 = VISA Close(VISA resource name=w1953, error in (no error)=w1952) -> ()  [unwired: 1 out]
        n636 = VISA Close(VISA resource name=w1950, error in (no error)=w1951) -> ()  [unwired: 1 out]
        n637 = Merge Errors(w1962, w1963, w1965, w1947) -> (w1964:errorcluster)
        n638 = call <vilib>:"Simple Error Handler.vi"("error in (no error)"=w1964) -> ("error?"=w1955:bool)  [unwired: 1 in, 7 out]
        n639 = Stop(stop? (T)=w1955) -> ()
      }
    }
  }
